vi "Wind_Turbine.vi"() -> (5 "Plug in titles":string[](array[string]), 7 "Plug in values":string[](array[string]))   [LabVIEW 2013]
uses:
  <vilib>/Analysis/baseanly.llb/Mean (DBL).vi
  Globals/Meas_global.vi
  Globals/LDA_meas_global_1.vi
  <vilib>/Analysis/NI_AALBase.lvlib
  <vilib>/Analysis/NI_AALPro.lvlib
panel:
  in  "Time Shift":dbl
  out "X array":dbl[](array[numeric])
  out "WT Numbers":string[](array[string])
  out "WT Revolution Start times":dbl[](array[numeric])
  out "Laser Disp Index":i32
  out "Laser Phase lock index":i32
  out "Laser Status Index":i32
  out "L Status Phase lock index":i32
  in  "Tab Control":T1(tab)
  in  "Change Dem Voltages?":bool=TRUE
  in  "Allow large changes?":bool
  out "Turbine RPMs":cluster{i32[], "All WTs":dbl[]}(graph)
  out "All WTs":dbl[][](array[numeric]) format="%#.2g"
  out "Cross Chs":cluster{dbl[], dbl[]}[](graph)
  in  "Cross_Corr to Phase Lock":i32[](listbox)
  in  "Channel to Phase lock":i32[](listbox)
  in  "Turbine to Phase Lock to":u16(ring) items=["RV (WT1)"]
  out "Inst Channels":cluster{dbl[], dbl[]}[](graph)
  in  "Add Phase data to results file":bool
  in  "Save Phase averaged Profiles":bool
  in  "Output Directory":path
  in  "Separation Character":string="\t"
  in  "Angular Step":dbl=1.0
  in  "Precision":string
  out "Av Disp 1":dbl
  out "Av Disp 2":dbl
  out "Av Disp 3":dbl
  out "Av Variance 1":dbl
  out "Av Variance 2":dbl
  out "Av Variance 3":dbl
  out "Angle 1":dbl format="%#_3g"
  out "Angle 2":dbl format="%#_3g"
  out "Angle 3":dbl format="%#_3g"
  out "Mean Blade 1":cluster{dbl, "Angular Step":dbl, dbl[]}(graph)
  out "slope 1":dbl format="%#_3g"
  out "Mean Blade 2":cluster{dbl, "Angular Step":dbl, dbl[]}(graph)
  out "Mean Blade 3":cluster{dbl, "Angular Step":dbl, dbl[]}(graph)
  out "slope 2":dbl format="%#_3g"
  out "slope 3":dbl format="%#_3g"
  out "Blade Positions":dbl[][](graph)
  out "Blade Angles":dbl[][](graph)
  out "Blade 1 Every Pass":dbl[](graph)
  out "Blade 2 Every Pass":dbl[](graph)
  out "Blade 3 Every Pass":dbl[](graph)
  out "Blade Analysis":string[][](table)
  in  "End Cut Deg":dbl
  in  "Start Cut Deg":dbl
  # "Mean RPM      SD RPM           Max-Min"
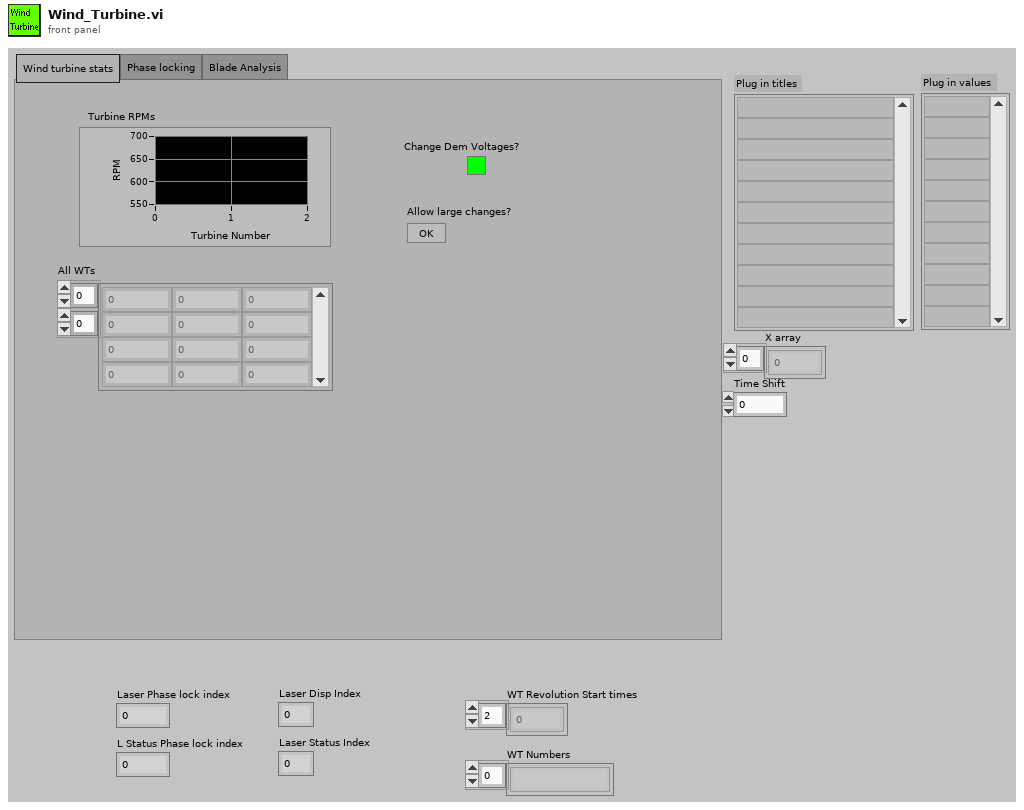
[diagram p1: front panel]
types:
  T1 = enum32{"Wind turbine stats", "Phase locking", "Blade Analysis"}
  T2 = typedef "Post_Process.ctl" = enum16{"Take New Data", "Post Process Raw Data File"}
  T3 = typedef "Analysis_info_cluster.ctl" = cluster{"Colour":u32, "Inst type":T4, "Inst name":string, "Symbol":string, "Code name":string, "Extra Info":string, "Inst Array":T5, "Extra Titles":string[], "Extra Values":string[], "U":dbl, "u^2":dbl, "u^3":dbl, "u^4":dbl, "Skew_u":dbl, "Kurt_u":dbl, "Sd Error in Mean":dbl, "% u'/U":dbl, "X":dbl, "Y":dbl, "Z":dbl, "Timescale integral to 25%":dbl, "Sd Error in Variance":dbl, "Calib File":path, "Calib Constants":dbl[], "Output Position":bool, "Full Stats":bool, "Av Sampling Rate":dbl, "Av No of Samples":dbl, "Total Meas Time (s)":dbl, "ADAM Ch Name":string}
  T4 = typedef "Inst_type.ctl" = enum16{"Propeller anemometer", "Raw voltage", "Pressure Transducer", "Pitot-static tube", "Preston tube", "Hot wire", "Cross wire 1", "Cross wire 2", "Generic Linear", "Generic Polynomial", "Generic BackPoly", "Fast FID", "Thermocouple", "Cold wire", "Pulsed Wire", "LDA Vel", "LDA Tran time", "LDA Arr time"}
  T5 = typedef "Instrument_Array.ctl" = enum16{"PWA", "LDA", "Analogue"}
  T6 = typedef "Time_Trace_Cluster.ctl" = cluster{"Weighting":dbl[], "Time (s)":dbl[], "Voltage":dbl[], "Eng Values":dbl[]}
  T7 = cluster{"X array":dbl[], "Phase locked uw/u'w'":dbl[]}
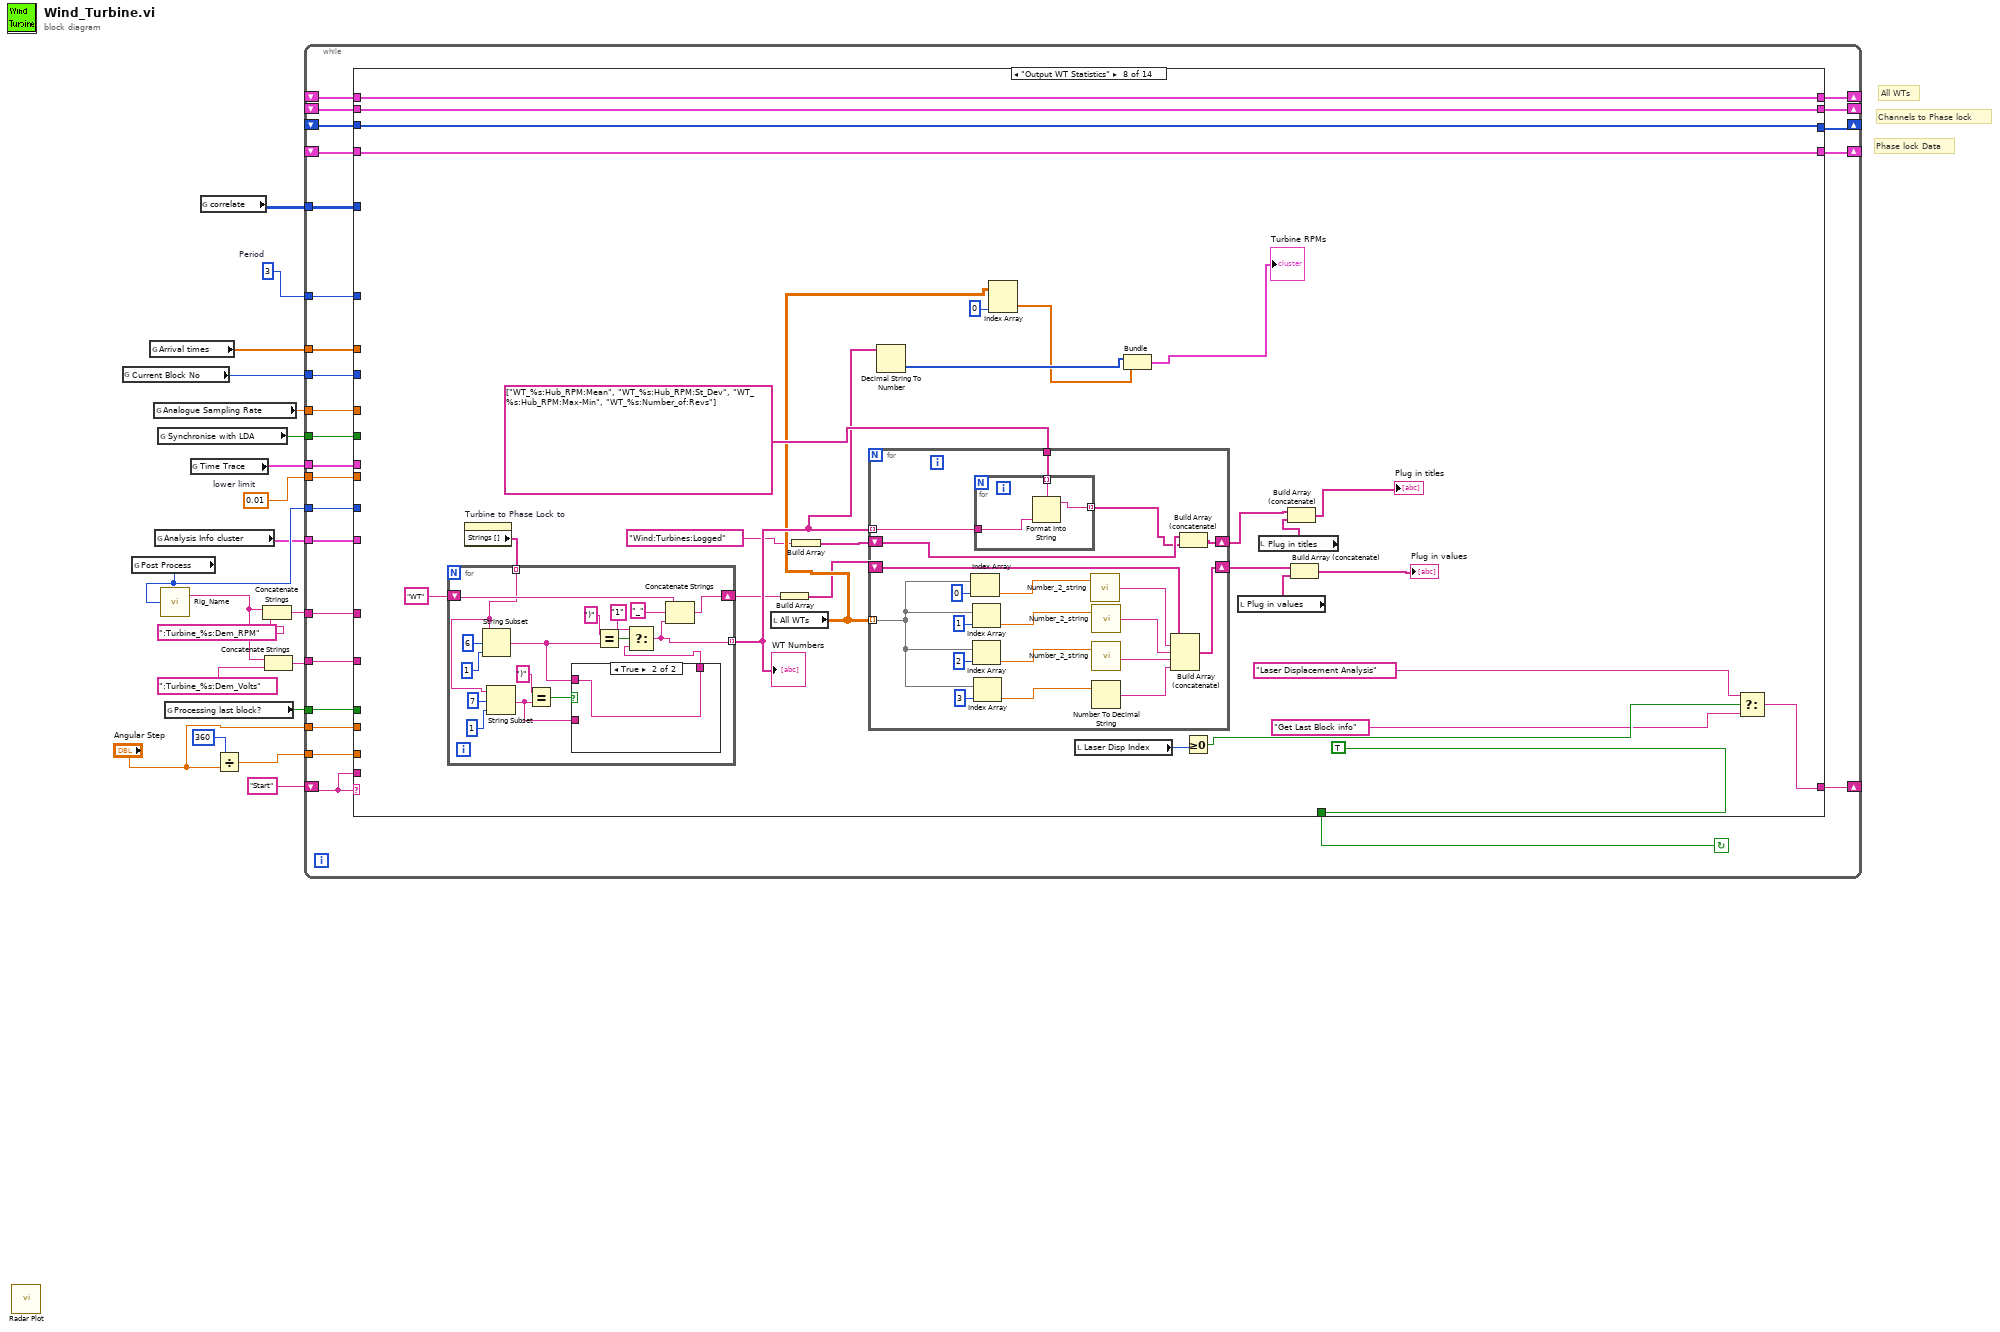
[diagram p0: block diagram]
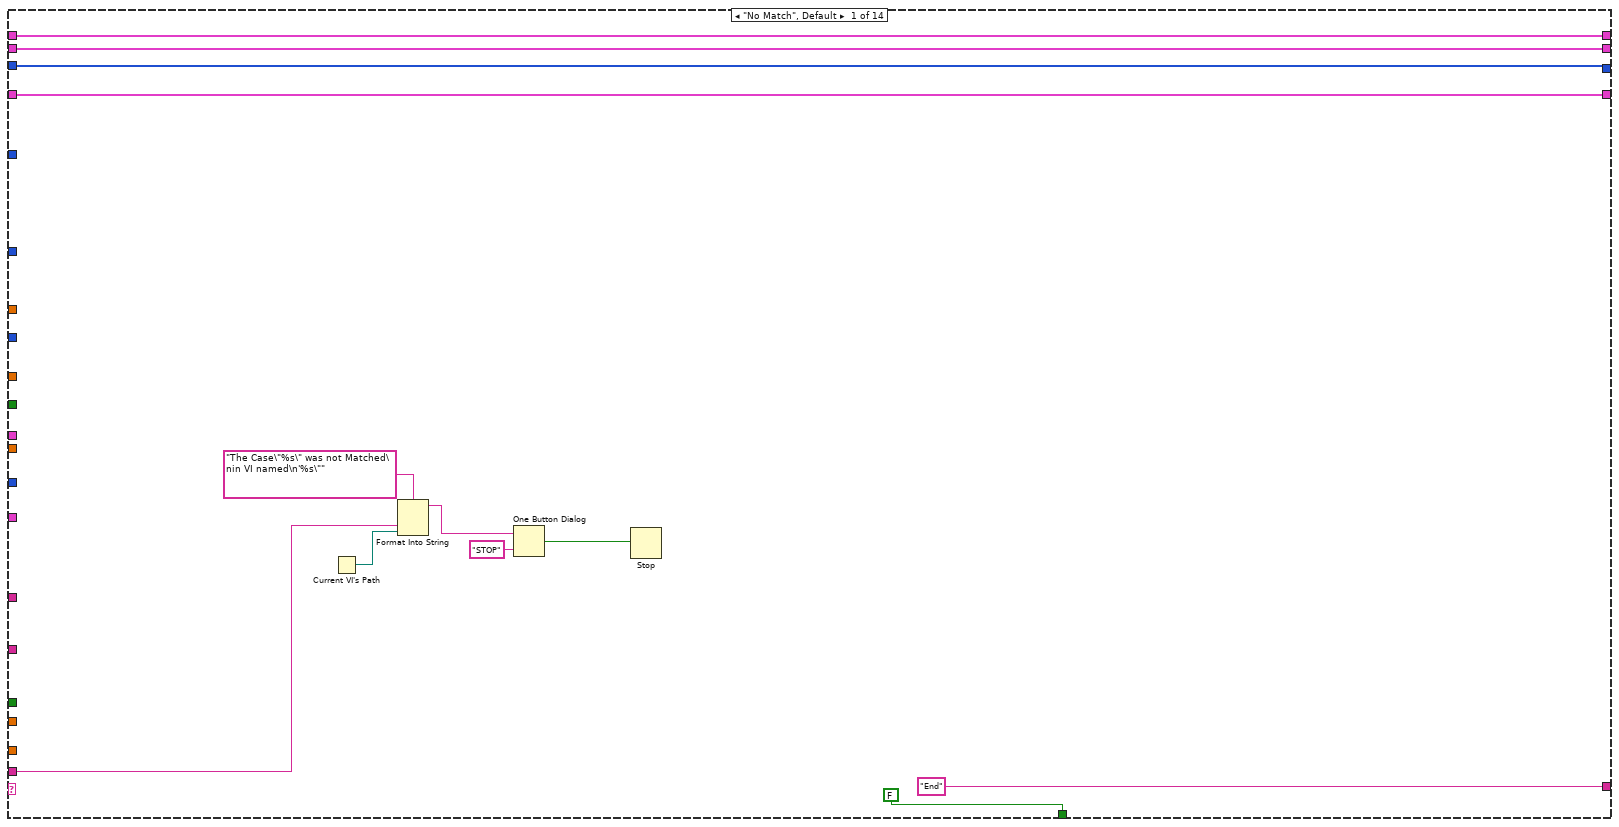
[diagram p2: hidden frame]
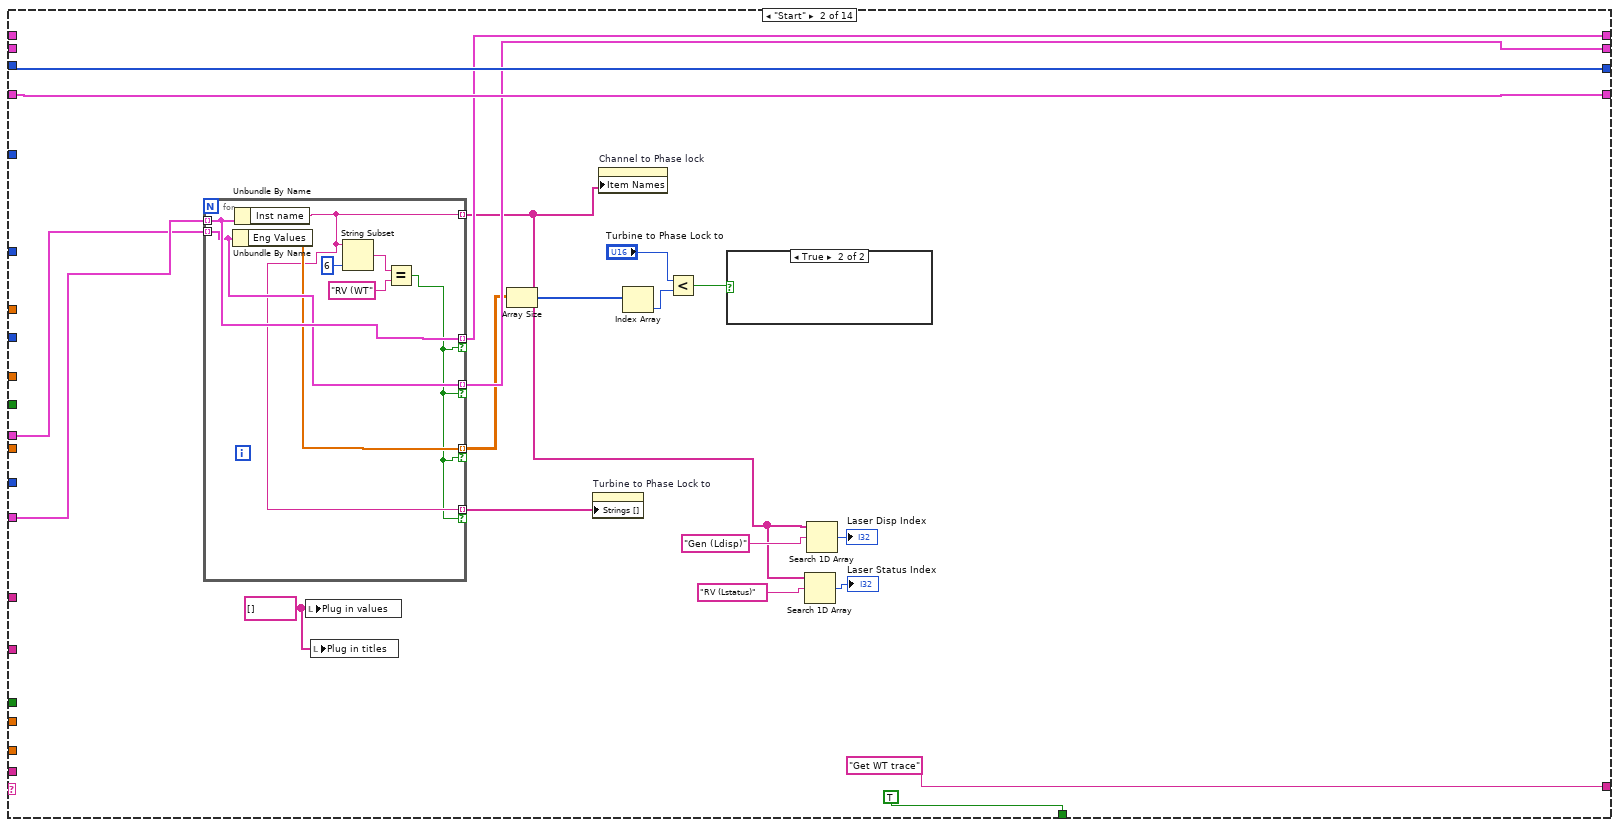
[diagram p3: hidden frame]
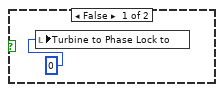
[diagram p4: hidden frame]
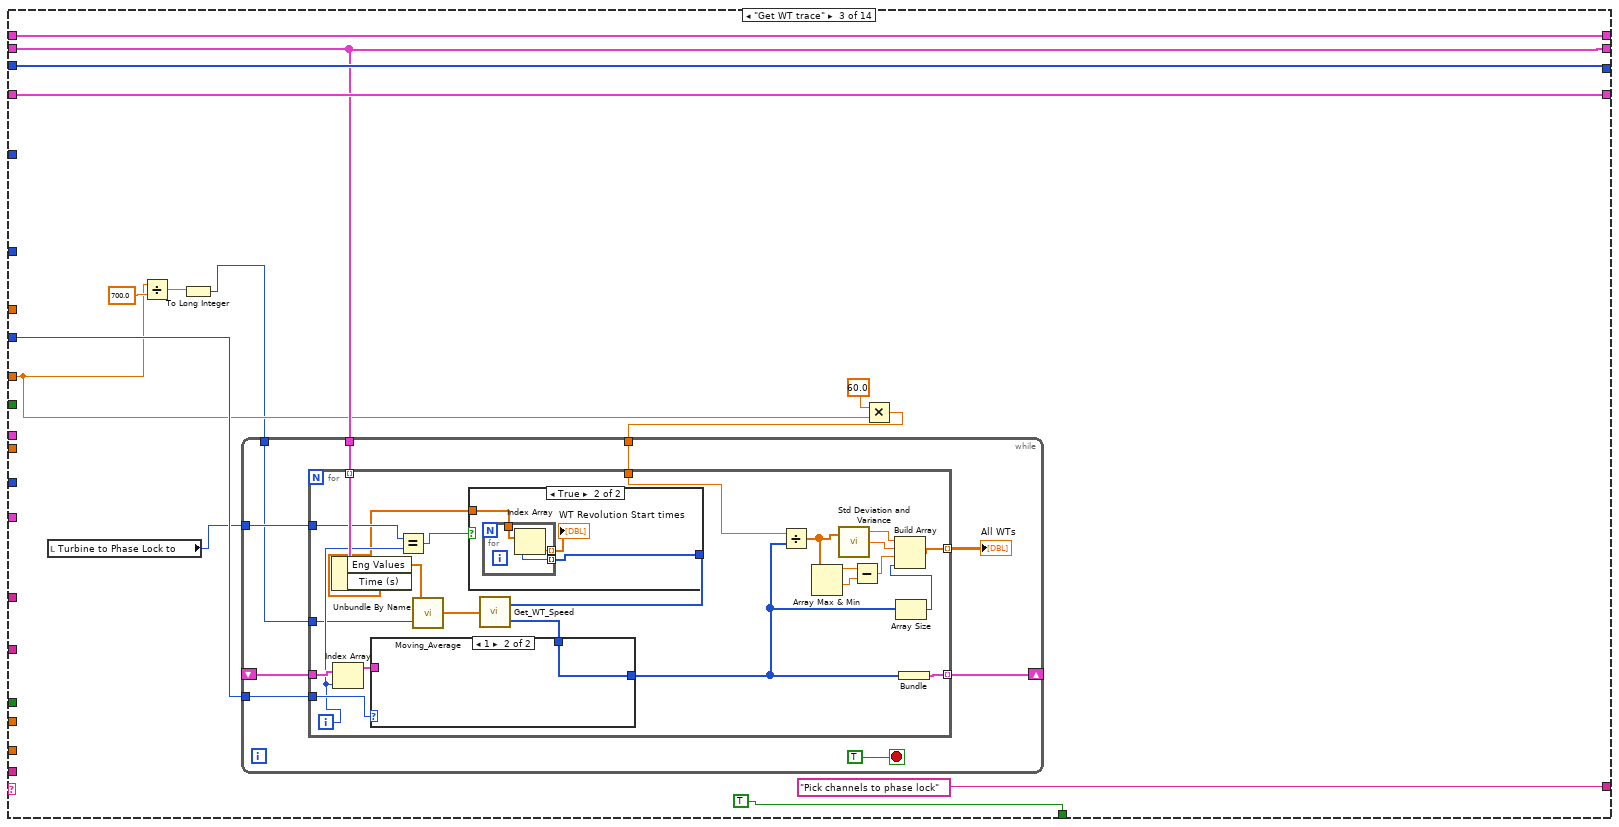
[diagram p5: hidden frame]
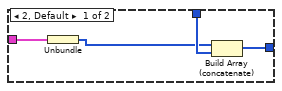
[diagram p7: hidden frame]
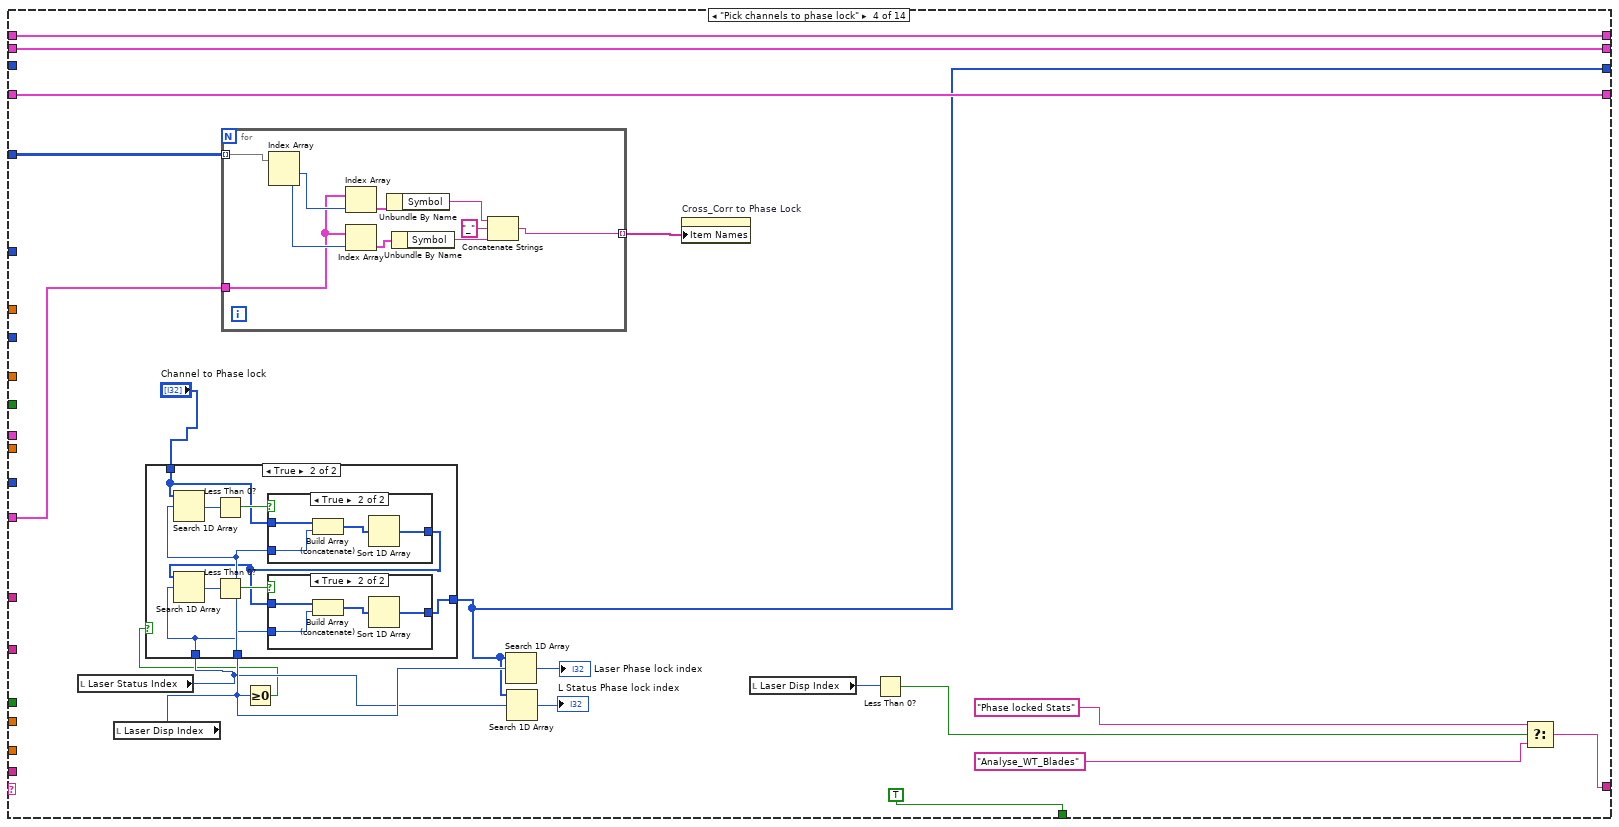
[diagram p8: hidden frame]
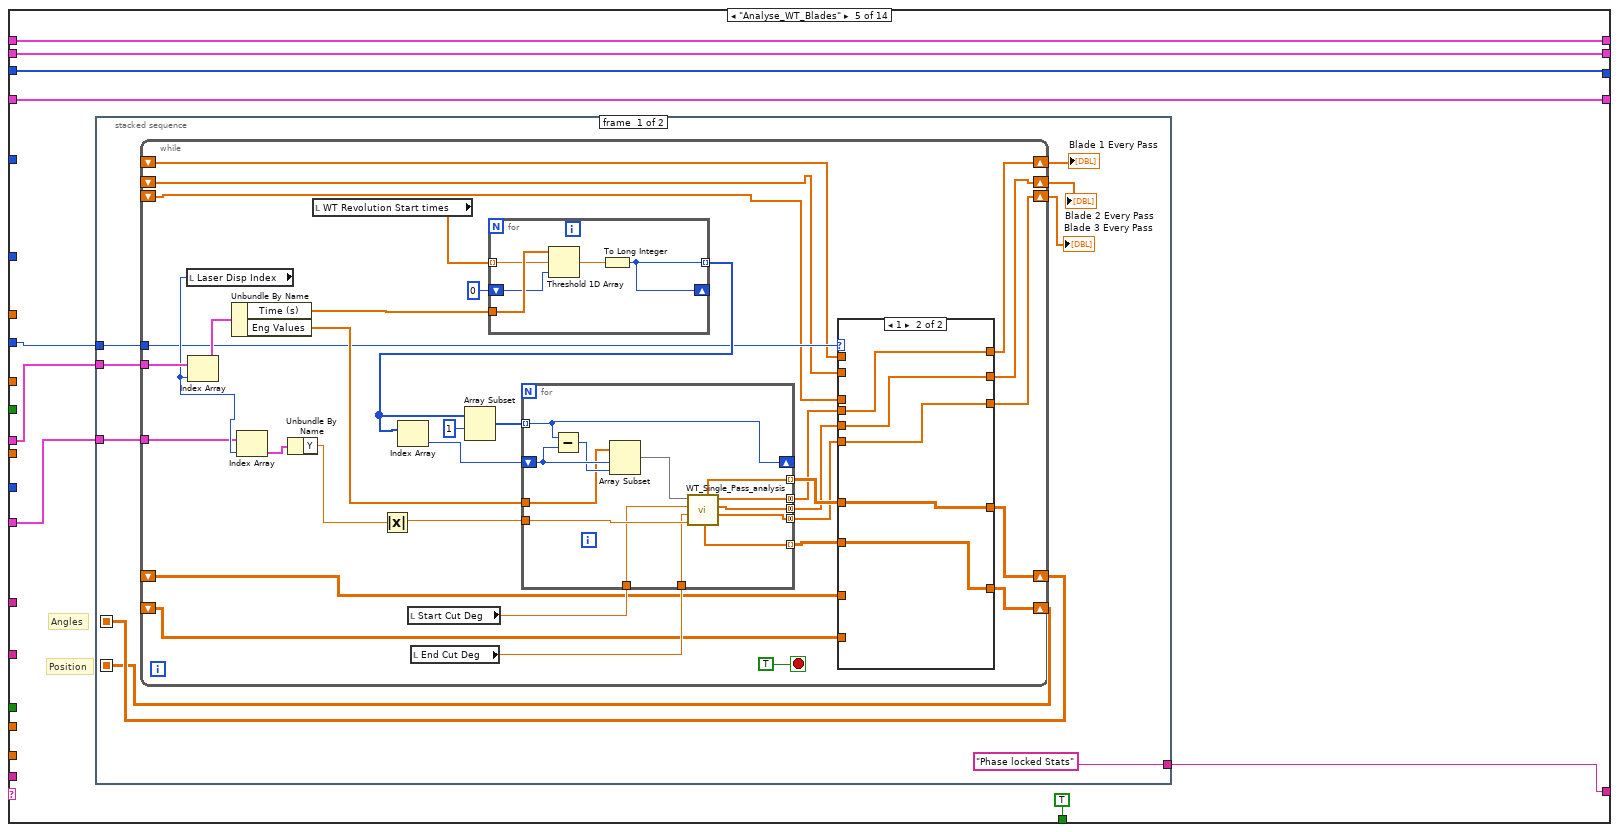
[diagram p12: hidden frame]
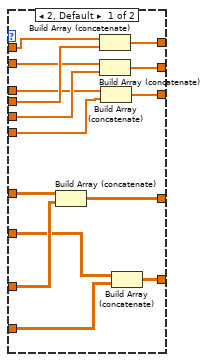
[diagram p13: hidden frame]
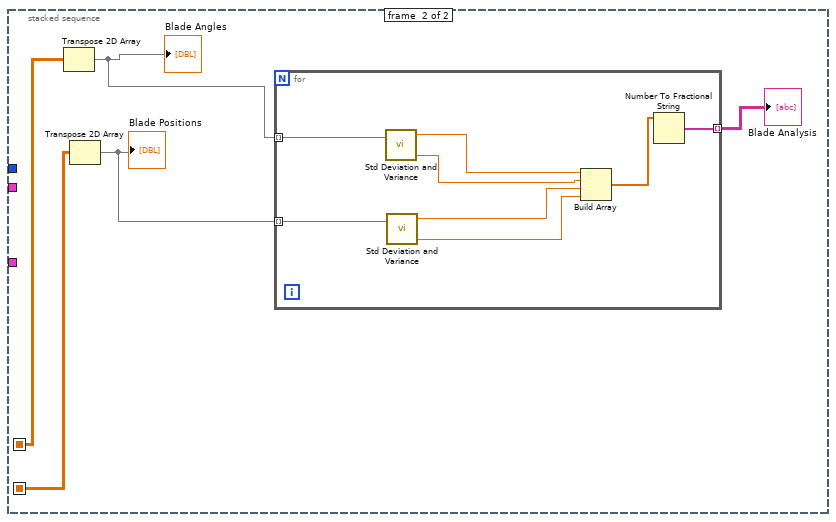
[diagram p14: hidden frame]
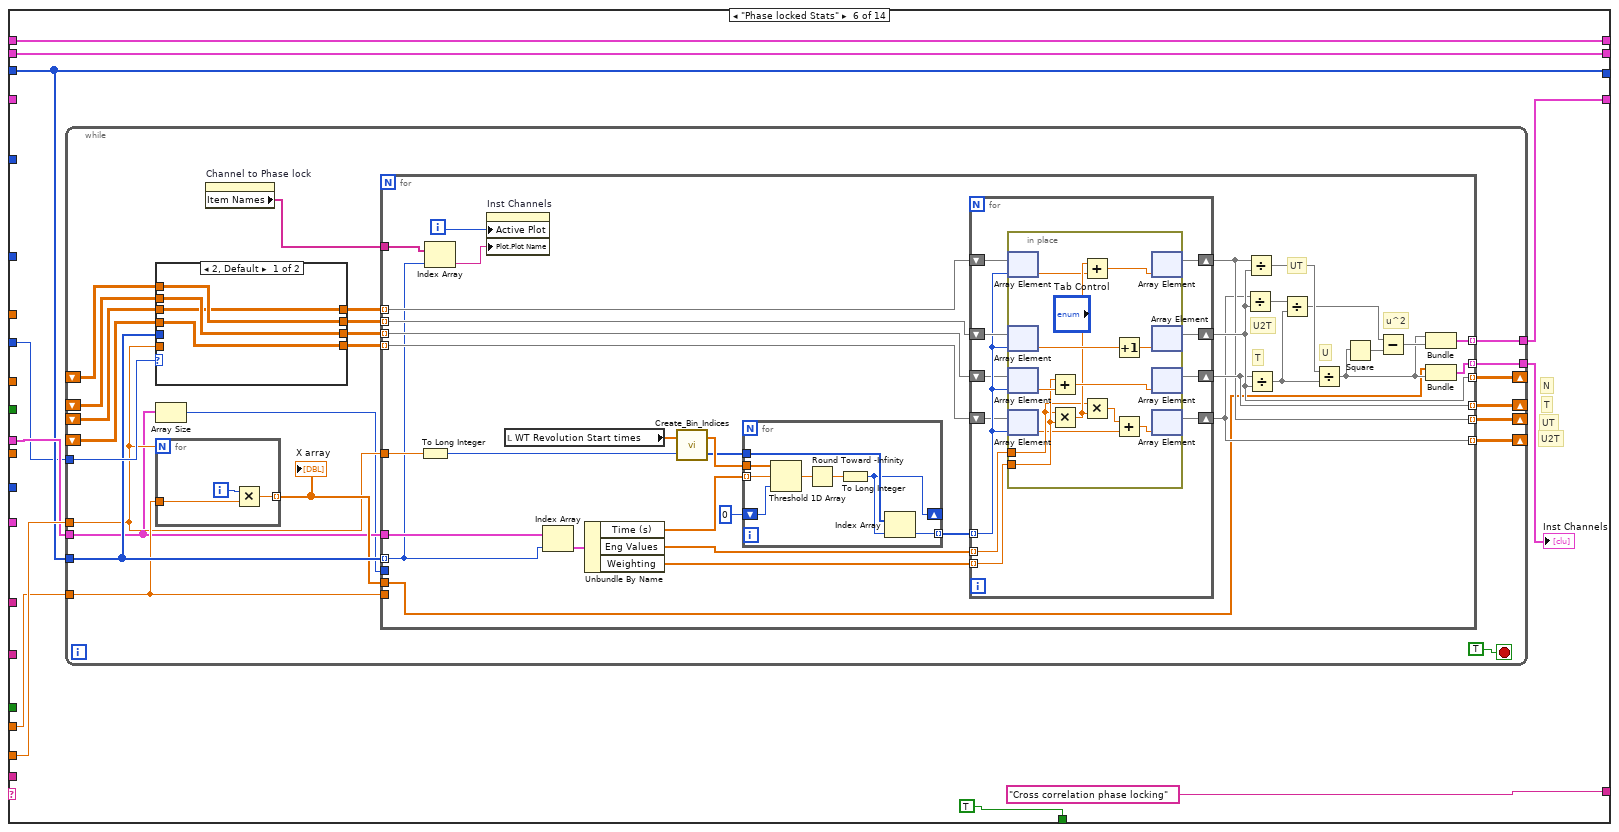
[diagram p15: hidden frame]
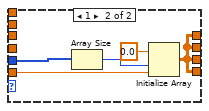
[diagram p16: hidden frame]
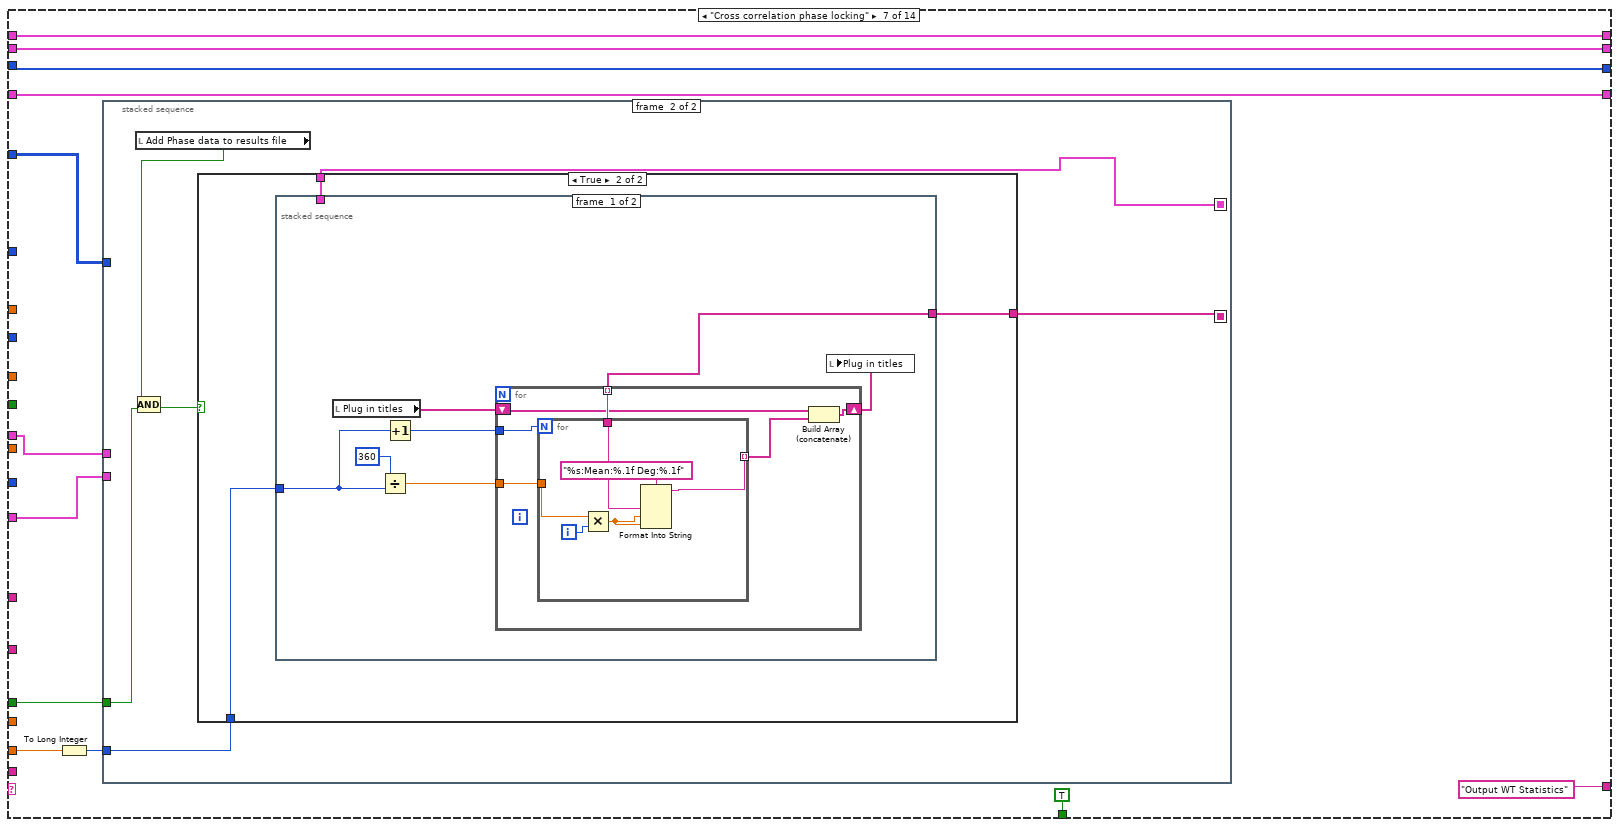
[diagram p17: hidden frame]
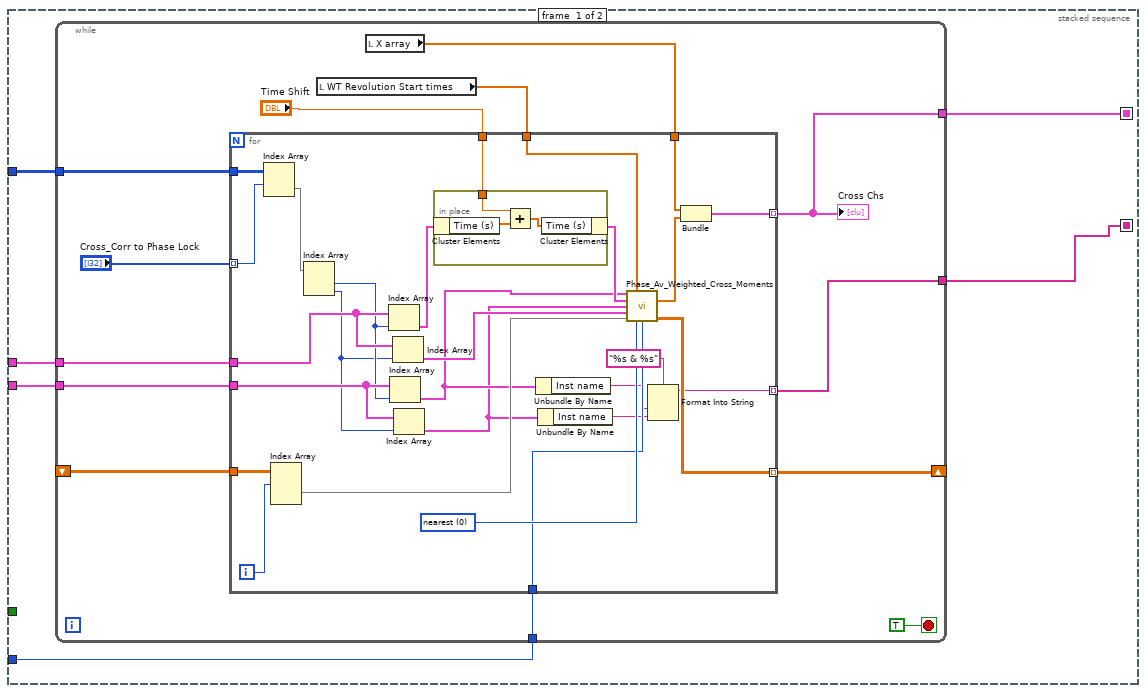
[diagram p18: hidden frame]
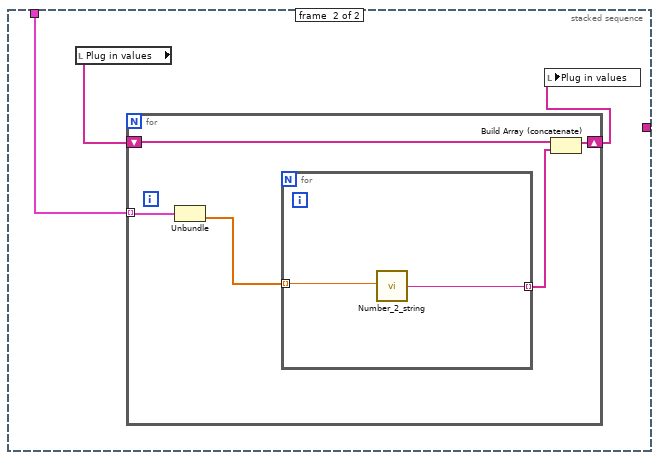
[diagram p20: hidden frame]
diagram:
  w18 = 3  # Period
  w19 = 0.01  # lower limit
  # "Phase lock Data"
  # "Channels to Phase lock"
  # "All WTs"
  n1 = call <vilib>:"Radar Plot.vi"() -> ()  [unwired: 15 in, 1 out]
  n2 = global read "Meas_global.vi" "Current Block No"() -> (w5:i32)
  n3 = global read "Meas_global.vi" "Post Process"() -> (w17:T2)
  n4 = global read "LDA_meas_global_1.vi" "Arrival times"() -> (w8:dbl[])
  n5 = global read "Meas_global.vi" "Analogue Sampling Rate"() -> (w20:dbl)
  n6 = global read "Meas_global.vi" "Analysis Info cluster"() -> (w7:T3[])
  n7 = global read "Meas_global.vi" "Synchronise with LDA"() -> (w12:bool)
  n8 = call "Rig_Name.vi"("Post Process"=w17) -> ("Rig Setup before dash"=w14:string)  [unwired: 1 out]
  n9 = global read "Meas_global.vi" "Processing last block?"() -> (w10:bool)
  n10 = global read "Meas_global.vi" "Time Trace"() -> (w3:T6[])
  n11 = global read "Meas_global.vi" "correlate"() -> (w1:i32[][])
  n12 = Divide(x=360, y="Angular Step") -> (x/y=w6:dbl)
  n13 = Concatenate Strings(w14, ":Turbine_%s:Dem_RPM") -> (w13:string)
  n14 = Concatenate Strings(w14, ":Turbine_%s:Dem_Volts") -> (w16:string)
  n15 = while {
    tunnel: w5 -> [w46]
    tunnel: w20 -> [w45]
    tunnel: w16 -> [w44]
    tunnel: w13 -> [w43]
    tunnel: w19 -> [w42]
    tunnel: w18 -> [w41]
    tunnel: w17 -> [w40]
    tunnel: w12 -> [w39]
    tunnel: w7 -> [w38]
    shift-right: [w22] -> _
    shift-left: "Start" -> [w36]
    tunnel: w10 -> [w35]
    tunnel: w6 -> [w34]
    tunnel: w8 -> [w33]
    tunnel: "Angular Step" -> [w32]
    shift-right: [w31] -> _
    shift-left: _ -> [w30]
    shift-right: [w28] -> _
    shift-left: _ -> [w29]
    shift-right: [w27] -> _
    shift-left: _ -> [w26]
    tunnel: w3 -> [w25]
    shift-right: [w24] -> _
    shift-left: _ -> [w23]
    tunnel: w1 -> [w21]
    stop <- w37 continue-if-true
    n16 = case shown="\"Output WT Statistics\"" w36 {
      tunnel: w46 -> [_ _ w97 _ w196 w301 _ _ _ _ _ _ _ _]
      tunnel: w45 -> [_ _ w90 _ _ _ _ _ w591 _ _ _ _ w975]
      tunnel: w44 -> [_ _ _ _ _ _ _ _ _ _ w865 _ _ _]
      tunnel: w43 -> [_ _ _ _ _ _ _ _ _ _ w840 _ _ _]
      tunnel: w42 -> [_ _ _ _ _ _ _ _ _ _ _ _ _ _]
      tunnel: w41 -> [_ _ _ _ _ _ _ _ _ _ _ _ _ _]
      tunnel: w40 -> [_ _ _ _ _ _ _ _ _ w825 _ _ _ _]
      tunnel: w39 -> [_ _ _ _ _ _ _ _ _ _ _ _ _ _]
      tunnel: w38 -> [_ w78 _ w148 w198 _ w412 _ w581 _ _ _ _ _]
      tunnel: ["End" "Get WT trace" "Pick channels to phase lock" w149 w195 "Cross correlation phase locking" "Output WT Statistics" w532 w586 w824 "End" ("f") "Check Folder Name" "Save Phase locked data" "End"] -> w22
      tunnel: [FALSE ("Change Control Voltage?") TRUE ("Processing last block?") TRUE TRUE ("Change Control Voltage?") TRUE ("Change Control Voltage?") TRUE TRUE ("Change Control Voltage?") TRUE ("Change Control Voltage?") w587 w823 FALSE ("Change Control Voltage?") w901 w952 FALSE ("Change Control Voltage?")] -> w37
      tunnel: w36 -> [w53 _ _ _ _ _ _ _ _ _ _ _ _ _]
      tunnel: w35 -> [_ _ _ _ _ _ w409 _ w588 w822 _ w899 _ _]
      tunnel: w34 -> [_ _ _ _ _ w308 w411 _ w590 _ _ w897 _ _]
      tunnel: w33 -> [_ _ _ _ _ _ _ _ _ _ _ _ _ _]
      tunnel: w32 -> [_ _ _ _ _ w307 _ _ w589 _ _ _ _ w969]
      tunnel: [w50 w64 w93 w164 w203 w306 w418 w529 w585 w821 w839 w896 w950 w972] -> w31
      tunnel: w30 -> [w50 _ w93 w164 w203 w306 w418 w529 w585 w821 w839 w896 w950 w972]
      tunnel: w29 -> [w49 w65 w95 _ w201 w302 w416 w528 w584 w820 w838 w895 w949 w971]
      tunnel: [w49 w65 w95 w155 w201 w302 w416 w528 w584 w820 w838 w895 w949 w971] -> w28
      tunnel: [w48 w66 w94 w159 w200 w300 w415 w527 w582 w819 w837 w893 w948 w970] -> w27
      tunnel: w26 -> [w48 w66 w94 w159 w200 _ w415 w527 w582 w819 w837 w893 w948 w970]
      tunnel: w25 -> [_ w67 _ _ w199 w303 w413 _ _ _ _ _ _ _]
      tunnel: [w47 w63 w92 w158 w202 w304 w417 w526 w583 w818 w836 w894 w947 w968] -> w24
      tunnel: w23 -> [w47 _ w92 w158 w202 w304 w417 w526 w583 w818 w836 w894 w947 w968]
      tunnel: w21 -> [_ _ _ w146 _ _ w414 _ _ _ _ _ _ _]
      frame "No Match", Default {
        n17 = Current VI's Path() -> (path=w54:path)
        n18 = Format Into String(format string="The Case\"%s\" was not Matched\nin VI named\n'%s\"" ("Format String"), w53, w54) -> (resulting string=w57:string)  [unwired: 2 in, 1 out]
        n19 = One Button Dialog(message=w57, button name ("OK")="STOP") -> (true=w55:bool)
        n20 = Stop(stop? (T)=w55) -> ()
      }
      frame "Start" {
        w59 = string[] [] ("Plug in values")
        n21 = for {
          tunnel: w78 -> [w84] mode=indexing
          tunnel: [w81] -> w60 mode=indexing
          tunnel: w67 -> [w83] mode=indexing
          tunnel: [w84] -> w64 mode=indexing if=w80
          tunnel: [w83] -> w63 mode=indexing if=w80
          tunnel: [w82] -> w62 mode=indexing if=w80
          tunnel: [w81] -> w61 mode=indexing if=w80
          n22 = Unbundle By Name(w83) -> ("Eng Values"=w82:dbl[])
          n23 = Unbundle By Name(w84) -> ("Inst name"=w81:string)
          n24 = String Subset(string=w81, length (rest)=6 ("length (rest)")) -> (substring=w85:string)  [unwired: 1 out]
          n25 = Equal?(x=w85, y="RV (WT") -> (x = y?=w80:bool)
        }
        n26 = local write "Plug in values"(w59) -> ()
        n27 = local write "Plug in titles"(w59) -> ()
        n28 = Array Size(array=w62) -> (size(s)=w69:i32[])
        n29 = property on="Turbine to Phase Lock to" class="Ring (strict)"("Strings []"=w61) -> ()  [unwired: 2 in, 2 out]
        n30 = property on="Channel to Phase lock" class="LstBox (strict)"("Item Names"=w60) -> ()  [unwired: 2 in, 2 out]
        n31 = Index Array(array=w69) -> (element=w68:i32)  [unwired: 1 in]
        n32 = Less?(x="Turbine to Phase Lock to", y=w68) -> (x < y?=w74:bool)
        n33 = case shown="True" w74 {
          frame False {
            n34 = local write "Turbine to Phase Lock to"(0) -> ()
          }
          frame True {
          }
        }
        n35 = Search 1D Array(1D array=w60, element="RV (Lstatus)") -> (index of element=→"Laser Status Index":i32)  [unwired: 1 in]
        n36 = Search 1D Array(1D array=w60, element="Gen (Ldisp)") -> (index of element=→"Laser Disp Index":i32)  [unwired: 1 in]
      }
      frame "Get WT trace" {
        n37 = local read "Turbine to Phase Lock to"() -> (w96:u16)
        n38 = Divide(x=w90, y=700.0) -> (x/y=w89:dbl)
        n39 = To Long Integer(number=w89) -> (32bit integer=w88:i32)
        n40 = Multiply(x=60.0, y=w90) -> (x*y=w98:dbl)
        n41 = while {
          tunnel: w97 -> [w110]
          shift-right: [w105] -> _
          shift-left: _ -> [w109]
          tunnel: w98 -> [w108]
          tunnel: w92 -> [w104]
          tunnel: w96 -> [w103]
          tunnel: w88 -> [w102]
          stop <- TRUE stop-if-true
          n42 = for {
            tunnel: w110 -> [w133]
            tunnel: w109 -> [w123]
            tunnel: w108 -> [w131]
            tunnel: [w124] -> w106 mode=indexing
            tunnel: [w119] -> w105 mode=indexing
            tunnel: w104 -> [w118] mode=indexing
            tunnel: w103 -> [w114]
            tunnel: w102 -> [w111]
            i -> [w115]
            n43 = Unbundle By Name(w118) -> ("Eng Values"=w117:dbl[], "Time (s)"=w112:dbl[])
            n44 = Index Array(array=w123, index=w115) -> (element=w122:cluster{"Samples per pulse":i32[]})
            n45 = Equal?(x=w114, y=w115) -> (x = y?=w113:bool)
            n46 = call "Moving_Average.vi"("Period"=w111, "Input Array"=w117) -> ("N+1-Period"=w134:dbl[])
            n47 = call "Get_WT_Speed.vi"("Opto Trace"=w134) -> ("Start Cycle Index"=w116:i32[], "Samples per pulse"=w132:i32[])
            n48 = case shown="1" w133 {
              tunnel: [w143 w145] -> w120
              tunnel: w132 -> [w144 w145]
              tunnel: w122 -> [w142 _]
              frame 2, Default {
                n49 = Unbundle(w142) -> ("Samples per pulse"=w141:i32[])
                n50 = Build Array (concatenate)(w141, w144) -> (w143:i32[])
              }
              frame 1 {
              }
            }
            n51 = case shown="True" w113 {
              tunnel: w116 -> [_ w137]
              tunnel: w112 -> [_ w136]
              frame False {
              }
              frame True {
                n52 = for {
                  tunnel: w137 -> [w140] mode=indexing
                  tunnel: w136 -> [w139]
                  tunnel: [w138] -> w135 mode=indexing
                  n53 = Index Array(array=w139, index=w140) -> (element=w138:dbl)
                }
                "WT Revolution Start times" <- w135
              }
            }
            n54 = Divide(x=w131, y=w120) -> (x/y=w128:dbl[])
            n55 = Array Max & Min(array=w128) -> (max value=w130:dbl, min value=w129:dbl)  [unwired: 2 out]
            n56 = call <vilib>:"Std Deviation and Variance.vi"("X"=w128) -> ("mean"=w127:dbl, "standard deviation"=w126:dbl)  [unwired: 1 in, 1 out]
            n57 = Subtract(x=w130, y=w129) -> (x-y=w125:dbl)
            n58 = Array Size(array=w120) -> (size(s)=w121:i32)
            n59 = Build Array(w127, w126, w125, w121) -> (w124:dbl[])
            n60 = Bundle("Samples per pulse"=w120) -> (w119:cluster{"Samples per pulse":i32[]})  [unwired: 1 in]
          }
          "All WTs" <- w106
        }
      }
      frame "Pick channels to phase lock" {
        n61 = local read "Laser Status Index"() -> (w161:i32)
        n62 = local read "Laser Disp Index"() -> (w162:i32)
        n63 = for {
          tunnel: w146 -> [w174] mode=indexing
          tunnel: w148 -> [w171]
          tunnel: [w165] -> w147 mode=indexing
          n64 = Index Array(array=w174) -> (element #1=w173:i32, element #2=w172:i32)  [unwired: 2 in]
          n65 = Index Array(array=w171, index=w173) -> (element=w170:T3)
          n66 = Index Array(array=w171, index=w172) -> (element=w169:T3)
          n67 = Unbundle By Name(w170) -> ("Symbol"=w168:string)
          n68 = Unbundle By Name(w169) -> ("Symbol"=w167:string)
          n69 = Concatenate Strings(w168, "_" ("string"), w167) -> (w165:string)
        }
        n70 = Greater Or Equal To 0?(x=w162) -> (x >= 0?=w160:bool)
        n71 = case shown="True" w160 {
          tunnel: "Channel to Phase lock" -> [w175 w182]
          tunnel: w162 -> [_ w181]
          tunnel: [w175 w178] -> w155
          tunnel: w161 -> [_ w176]
          frame False {
          }
          frame True {
            n72 = Search 1D Array(1D array=w182, element=w181) -> (index of element=w184:i32)  [unwired: 1 in]
            n73 = Less Than 0?(x=w184) -> (x < 0?=w183:bool)
            n74 = case shown="True" w183 {
              tunnel: w182 -> [w190 w194]
              tunnel: w181 -> [_ w193]
              tunnel: [w190 w191] -> w177
              frame False {
              }
              frame True {
                n75 = Build Array (concatenate)(w194, w193) -> (w192:i32[])
                n76 = Sort 1D Array(array=w192) -> (sorted array=w191:i32[])
              }
            }
            n77 = Search 1D Array(1D array=w177, element=w176) -> (index of element=w179:i32)  [unwired: 1 in]
            n78 = Less Than 0?(x=w179) -> (x < 0?=w180:bool)
            n79 = case shown="True" w180 {
              tunnel: w177 -> [w185 w189]
              tunnel: w176 -> [_ w188]
              tunnel: [w185 w186] -> w178
              frame False {
              }
              frame True {
                n80 = Build Array (concatenate)(w189, w188) -> (w187:i32[])
                n81 = Sort 1D Array(array=w187) -> (sorted array=w186:i32[])
              }
            }
          }
        }
        n82 = Search 1D Array(1D array=w155, element=w162) -> (index of element=→"Laser Phase lock index":i32)  [unwired: 1 in]
        n83 = Search 1D Array(1D array=w155, element=w161) -> (index of element=→"L Status Phase lock index":i32)  [unwired: 1 in]
        n84 = property on="Cross_Corr to Phase Lock" class="LstBox (strict)"("Item Names"=w147) -> ()  [unwired: 2 in, 2 out]
        n85 = local read "Laser Disp Index"() -> (w153:i32)
        n86 = Less Than 0?(x=w153) -> (x < 0?=w152:bool)
        n87 = Select(t="Phase locked Stats" ("f"), s=w152, f="Analyse_WT_Blades") -> (s? t:f=w149:string)
      }
      frame "Analyse_WT_Blades" {
        # "Position"
        # "Angles"
        n88 = stacked-sequence {
          seq-local: [w207 _] -> [_ w288]
          seq-local: [w208 _] -> [_ w289]
          tunnel: w199 -> [w212 _]
          tunnel: w198 -> [w211 _]
          tunnel: w196 -> [w210 _]
          tunnel: ["Phase locked Stats" ("f") _] -> w195
          frame #0 {
            n89 = while {
              tunnel: w212 -> [w246]
              tunnel: w211 -> [w235]
              shift-right: [w225] -> w208
              shift-left: _ -> [w226]
              shift-right: [w222] -> w207
              shift-left: _ -> [w223]
              tunnel: w210 -> [w228]
              shift-right: [w220] -> w206
              shift-left: _ -> [w219]
              shift-right: [w215] -> w205
              shift-left: _ -> [w216]
              shift-right: [w213] -> w204
              shift-left: _ -> [w214]
              stop <- TRUE stop-if-true
              n90 = local read "Laser Disp Index"() -> (w236:i32)
              n91 = Index Array(array=w246, index=w236) -> (element=w245:T6)
              n92 = Unbundle By Name(w245) -> ("Time (s)"=w244:dbl[], "Eng Values"=w237:dbl[])
              n93 = Index Array(array=w235, index=w236) -> (element=w234:T3)
              n94 = Unbundle By Name(w234) -> ("Y"=w233:dbl)
              n95 = local read "WT Revolution Start times"() -> (w243:dbl[])
              n96 = Absolute Value(x=w233) -> (abs(x)=w232:dbl)
              n97 = local read "Start Cut Deg"() -> (w231:dbl)
              n98 = local read "End Cut Deg"() -> (w230:dbl)
              n99 = for {
                tunnel: w244 -> [w284]
                tunnel: w243 -> [w283] mode=indexing
                shift-right: [w280] -> _
                shift-left: 0 -> [w282]
                tunnel: [w280] -> w240 mode=indexing
                n100 = Threshold 1D Array(1:w282, 2:w283, 3:w284) -> (0:w281:dbl)
                n101 = To Long Integer(number=w281) -> (32bit integer=w280:i32)
              }
              n102 = Index Array(array=w240) -> (element=w239:i32)  [unwired: 1 in]
              n103 = Array Subset(array=w240, index=1) -> (w238:i32[])  [unwired: 1 in]
              n104 = for {
                shift-right: [w278] -> _
                shift-left: w239 -> [w279]
                tunnel: w238 -> [w278] mode=indexing
                tunnel: w237 -> [w276]
                tunnel: w232 -> [w274]
                tunnel: [w270] -> w227 mode=indexing
                tunnel: [w273] -> w224 mode=indexing
                tunnel: w231 -> [w272]
                tunnel: w230 -> [w271]
                tunnel: [w269] -> w221 mode=concatenating
                tunnel: [w268] -> w218 mode=concatenating
                tunnel: [w267] -> w217 mode=concatenating
                n105 = Subtract(x=w278, y=w279) -> (x-y=w277:i32)
                n106 = Array Subset(array=w276, index=w279, length=w277) -> (w275:dbl[])
                n107 = call "WT_Single_Pass_analysis.vi"("Displacement"=w275, "Start Cut Deg"=w272, "End Cut Deg"=w271, "Radius"=w274) -> ("Blade Angles"=w270:dbl[], "Blade Positions"=w273:dbl[], "Blade1"=w269:dbl[], "Blade 2"=w268:dbl[], "Blade 3"=w267:dbl[])  [unwired: 1 in]
              }
              n108 = case shown="1" w228 {
                tunnel: w227 -> [w261 w266]
                tunnel: w226 -> [w260 _]
                tunnel: [w259 w266] -> w225
                tunnel: w224 -> [w258 w265]
                tunnel: w223 -> [w257 _]
                tunnel: [w256 w265] -> w222
                tunnel: w221 -> [w255 w264]
                tunnel: [w253 w264] -> w220
                tunnel: w219 -> [w254 _]
                tunnel: w218 -> [w252 w263]
                tunnel: w217 -> [w251 w262]
                tunnel: w216 -> [w250 _]
                tunnel: [w249 w263] -> w215
                tunnel: w214 -> [w248 _]
                tunnel: [w247 w262] -> w213
                frame 2, Default {
                  n109 = Build Array (concatenate)(w261, w260) -> (w259:dbl[][])
                  n110 = Build Array (concatenate)(w254, w255) -> (w253:dbl[])
                  n111 = Build Array (concatenate)(w250, w252) -> (w249:dbl[])
                  n112 = Build Array (concatenate)(w248, w251) -> (w247:dbl[])
                  n113 = Build Array (concatenate)(w258, w257) -> (w256:dbl[][])
                }
                frame 1 {
                }
              }
            }
            "Blade 1 Every Pass" <- w206
            "Blade 3 Every Pass" <- w204
            "Blade 2 Every Pass" <- w205
          }
          frame #1 {
            n114 = Transpose 2D Array(2D array=w289) -> (transposed array=w286:dbl[][])
            "Blade Angles" <- w286
            n115 = Transpose 2D Array(2D array=w288) -> (transposed array=w287:dbl[][])
            "Blade Positions" <- w287
            n116 = for {
              tunnel: w286 -> [w297] mode=indexing
              tunnel: w287 -> [w296] mode=indexing
              tunnel: [w290] -> w285 mode=indexing
              n117 = call <vilib>:"Std Deviation and Variance.vi"("X"=w297) -> ("mean"=w295:dbl, "variance"=w294:dbl)  [unwired: 1 in, 1 out]
              n118 = call <vilib>:"Std Deviation and Variance.vi"("X"=w296) -> ("mean"=w293:dbl, "variance"=w292:dbl)  [unwired: 1 in, 1 out]
              n119 = Build Array(w295, w294, w293, w292) -> (w291:dbl[])
              n120 = Number To Fractional String(number=w291) -> (F-format string=w290:string[])  [unwired: 3 in]
            }
            "Blade Analysis" <- w285
          }
        }
      }
      frame "Phase locked Stats" {
        # "N"
        # "U2T"
        # "UT"
        # "T"
        n121 = while {
          tunnel: w308 -> [w312]
          tunnel: w307 -> [w314]
          tunnel: w302 -> [w329]
          shift-right: [w318] -> _
          shift-left: _ -> [w324]
          tunnel: w303 -> [w311]
          shift-right: [w317] -> _
          shift-left: _ -> [w323]
          shift-right: [w316] -> _
          shift-left: _ -> [w322]
          shift-right: [w315] -> _
          shift-left: _ -> [w321]
          tunnel: w301 -> [w330]
          tunnel: [w320] -> w300
          tunnel: [w319] -> w298
          stop <- TRUE stop-if-true
          n122 = case shown="2, Default" w330 {
            tunnel: w312 -> [_ w342]
            tunnel: w329 -> [_ w341]
            tunnel: [w338 w339] -> w328
            tunnel: [w337 w339] -> w327
            tunnel: [w336 w339] -> w326
            tunnel: [w335 w339] -> w325
            tunnel: w324 -> [w338 _]
            tunnel: w323 -> [w337 _]
            tunnel: w322 -> [w336 _]
            tunnel: w321 -> [w335 _]
            frame 2, Default {
            }
            frame 1 {
              n123 = Array Size(array=w341) -> (size(s)=w340:i32)
              n124 = Initialize Array(0.0, w340, w342) -> (w339:dbl[][])
            }
          }
          n125 = Array Size(array=w311) -> (size(s)=w310:i32)
          n126 = for {
            N: w312 -> [_]
            tunnel: w314 -> [w333]
            tunnel: [w332] -> w313 mode=indexing
            i -> [w334]
            n127 = Multiply(x=w334, y=w333) -> (x*y=w332:dbl)
          }
          "X array" <- w313
          n128 = property on="Channel to Phase lock" class="LstBox (strict)"() -> ("Item Names"=w309:string[])  [unwired: 2 in, 2 out]
          n129 = for {
            tunnel: w312 -> [w372]
            tunnel: w314 -> [_]
            tunnel: w329 -> [w345] mode=indexing
            tunnel: w311 -> [w368]
            tunnel: w328 -> [w357] mode=indexing
            tunnel: [w353] -> w318 mode=indexing
            tunnel: [w352] -> w317 mode=indexing
            tunnel: [w351] -> w316 mode=indexing
            tunnel: [w350] -> w315 mode=indexing
            tunnel: w327 -> [w356] mode=indexing
            tunnel: w326 -> [w355] mode=indexing
            tunnel: w325 -> [w354] mode=indexing
            tunnel: [w360] -> w320 mode=indexing
            tunnel: [w358] -> w319 mode=indexing
            tunnel: w313 -> [w349]
            tunnel: w310 -> [_]
            tunnel: w309 -> [w347]
            i -> [w348]
            # "u^2"
            # "U"
            # "U2T"
            # "UT"
            # "T"
            n130 = To Long Integer(number=w372) -> (32bit integer=w371:i32)
            n131 = Index Array(array=w347, index=w345) -> (element=w346:string)
            n132 = property on="Inst Channels" class="XYGraph (strict)"("Active Plot"=w348, "Plot.Plot Name"=w346) -> ()  [unwired: 2 in, 2 out]
            n133 = local read "WT Revolution Start times"() -> (w376:dbl[])
            n134 = Index Array(array=w368, index=w345) -> (element=w344:T6)
            n135 = Unbundle By Name(w344) -> ("Time (s)"=w370:dbl[], "Eng Values"=w369:dbl[], "Weighting"=w367:dbl[])
            n136 = call "Create_Bin_Indices.vi"("No Of Bins"=w371, "Cycle Start TIme"=w376) -> ("Bin Number"=w374:i32[], "Bin Start Time"=w375:dbl[])
            n137 = for {
              tunnel: w375 -> [w408]
              tunnel: w370 -> [w407] mode=indexing
              shift-right: [w404] -> _
              shift-left: 0 -> [w401]
              tunnel: w374 -> [w405]
              tunnel: [w403] -> w373 mode=indexing
              n138 = Threshold 1D Array(1:w401, 2:w407, 3:w408) -> (0:w406:dbl)
              n139 = Round Toward -Infinity(1:w406) -> (0:w402:dbl)
              n140 = To Long Integer(number=w402) -> (32bit integer=w404:i32)
              n141 = Index Array(array=w405, index=w404) -> (element=w403:i32)
            }
            n142 = for {
              tunnel: w373 -> [w387] mode=indexing
              tunnel: w369 -> [w379] mode=indexing
              tunnel: w367 -> [w378] mode=indexing
              shift-right: [w383] -> w353
              shift-left: w357 -> [w388]
              shift-right: [w382] -> w352
              shift-left: w356 -> [w384]
              shift-right: [w381] -> w351
              shift-left: w355 -> [w385]
              shift-right: [w380] -> w350
              shift-left: w354 -> [w386]
              n143 = in-place {
                in-place-border: w379 -> [w393]
                in-place-border: w378 -> [w396]
                n144 = in-place-array #1(w385, w387) -> (w390:dbl)
                n145 = in-place-array #2(w388, w387) -> (w400:dbl)
                n146 = in-place-array #3(w384, w387) -> (w398:dbl)
                n147 = in-place-array #4(w386, w387) -> (w389:dbl)
                n148 = Add(x=w396, y=w398) -> (x+y=w397:dbl)
                n149 = Multiply(x=w393, y=w396) -> (x*y=w395:dbl)
                n150 = Add(x=w395, y=w390) -> (x+y=w391:dbl)
                n151 = Multiply(x=w393, y=w395) -> (x*y=w394:dbl)
                n152 = Increment(x=w400) -> (x+1=w399:dbl)
                n153 = Add(x=w394, y=w389) -> (x+y=w392:dbl)
                n154 = in-place-array #1(w391) -> (w381:dbl[])  [unwired: 1 out]
                n155 = in-place-array #2(w399) -> (w383:dbl[])  [unwired: 1 out]
                n156 = in-place-array #3(w397) -> (w382:dbl[])  [unwired: 1 out]
                n157 = in-place-array #4(w392) -> (w380:dbl[])  [unwired: 1 out]
              }
            }
            n158 = Divide(x=w350, y=w353) -> (x/y=w364:dbl[])
            n159 = Divide(x=w351, y=w353) -> (x/y=w366:dbl[])
            n160 = Divide(x=w352, y=w353) -> (x/y=w365:dbl[])
            n161 = Divide(x=w364, y=w365) -> (x/y=w363:dbl[])
            n162 = Divide(x=w366, y=w365) -> (x/y=w359:dbl[])
            n163 = Square(x=w359) -> (x^2=w362:dbl[])
            n164 = Subtract(x=w363, y=w362) -> (x-y=w361:dbl[])
            n165 = Bundle(w359, w361) -> (w360:cluster{dbl[], dbl[]})  [unwired: 1 in]
            n166 = Bundle(w349, w359) -> (w358:cluster{dbl[], dbl[]})  [unwired: 1 in]
          }
        }
        "Inst Channels" <- w298
      }
      frame "Cross correlation phase locking" {
        n167 = To Long Integer(number=w411) -> (32bit integer=w410:i32)
        n168 = stacked-sequence {
          seq-local: [w422 _] -> [_ w475]
          seq-local: [w421 _] -> [_ w474]
          tunnel: w414 -> [w426 _]
          tunnel: w413 -> [w425 _]
          tunnel: w412 -> [w424 _]
          tunnel: w410 -> [w423 w473]
          tunnel: w409 -> [_ w470]
          frame #0 {
            n169 = while {
              shift-right: [w439] -> _
              shift-left: _ -> [w438]
              tunnel: w426 -> [w435]
              tunnel: w425 -> [w434]
              tunnel: w424 -> [w433]
              tunnel: w423 -> [w430]
              tunnel: [w428] -> w422
              tunnel: [w427] -> w421
              stop <- TRUE stop-if-true
              n170 = local read "WT Revolution Start times"() -> (w431:dbl[])
              n171 = local read "X array"() -> (w437:dbl[])
              n172 = for {
                tunnel: [w466] -> w439 mode=indexing
                tunnel: w438 -> [w465]
                tunnel: w437 -> [w462]
                tunnel: [w460] -> w428 mode=indexing
                tunnel: "Cross_Corr to Phase Lock" -> [w459] mode=indexing
                tunnel: w435 -> [w458]
                tunnel: w434 -> [w456]
                tunnel: w433 -> [w454]
                tunnel: w431 -> [w450]
                tunnel: w430 -> [w449]
                tunnel: "Time Shift" -> [w446]
                tunnel: [w440] -> w427 mode=indexing
                i -> [w464]
                w451 = 0 items=["nearest", "linear", "spline", "cubic Hermite", "Lagrange"] ("interp. method")
                n173 = Index Array(array=w458, index (row)=w459) -> (element=w457:i32[])  [unwired: 1 in]
                n174 = Index Array(array=w465, index (dim 0)=w464) -> (element=w463:dbl[][])  [unwired: 2 in]
                n175 = Index Array(array=w457) -> (element #1=w453:i32, element #2=w452:i32)  [unwired: 2 in]
                n176 = Index Array(array=w456, index=w453) -> (element=w448:T6)
                n177 = Index Array(array=w454, index=w453) -> (element=w445:T3)
                n178 = Index Array(array=w456, index=w452) -> (element=w455:T6)
                n179 = Index Array(array=w454, index=w452) -> (element=w444:T3)
                n180 = in-place {
                  in-place-border: w446 -> [w469]
                  n181 = in-place-cluster #5(w448) -> ("Time (s)"=w468:dbl[])
                  n182 = Add(x=w469, y=w468) -> (x+y=w467:dbl[])
                  n183 = in-place-cluster #5("Time (s)"=w467) -> (w447:T6)
                }
                n184 = Unbundle By Name(w445) -> ("Inst name"=w443:string)
                n185 = Unbundle By Name(w444) -> ("Inst name"=w442:string)
                n186 = call "Phase_Av_Weighted_Cross_Moments.vi"("AI Cluster 1"=w445, "WT Revolution Start times"=w450, "Time Cluster 1"=w447, "AI Cluster 2"=w444, "Time Cluster 2"=w455, "Shift in"=w463, "interp. method"=w451, "No Of Bins"=w449) -> ("Phase locked uw/u'w'"=w461:dbl[], "Shift out"=w466:dbl[][])  [unwired: 5 in, 1 out]
                n187 = Format Into String(format string="%s & %s", w443, w442) -> (resulting string=w440:string)  [unwired: 2 in, 1 out]
                n188 = Bundle("X array"=w462, "Phase locked uw/u'w'"=w461) -> (w460:T7)  [unwired: 1 in]
              }
              "Cross Chs" <- w428
            }
          }
          frame #1 {
            n189 = local read "Add Phase data to results file"() -> (w471:bool)
            n190 = Compound Arithmetic op=AND(w471, w470) -> (w472:bool)
            n191 = case shown="True" w472 {
              tunnel: w475 -> [_ w478]
              tunnel: w474 -> [_ w477]
              tunnel: w473 -> [_ w476]
              frame False {
              }
              frame True {
                n192 = stacked-sequence {
                  tunnel: w476 -> [w481 _]
                  tunnel: w478 -> [_ w498]
                  tunnel: w477 -> [w479 _]
                  frame #0 {
                    n193 = local read "Plug in titles"() -> (w482:string[])
                    n194 = Divide(x=360, y=w481) -> (x/y=w484:dbl)
                    n195 = Increment(x=w481) -> (x+1=w480:i32)
                    n196 = for {
                      tunnel: w479 -> [w491] mode=indexing
                      tunnel: w484 -> [w490]
                      shift-right: [w487] -> w483
                      shift-left: w482 -> [w489]
                      tunnel: w480 -> [w486]
                      n197 = for {
                        N: w486 -> [_]
                        tunnel: w491 -> [w493]
                        tunnel: w490 -> [w496]
                        tunnel: [w494] -> w488 mode=indexing
                        i -> [w497]
                        n198 = Multiply(x=w496, y=w497) -> (x*y=w492:dbl)
                        n199 = Format Into String(format string="%s:Mean:%.1f Deg:%.1f", w493, w492, w492) -> (resulting string=w494:string)  [unwired: 2 in, 1 out]
                      }
                      n200 = Build Array (concatenate)(w489, w488) -> (w487:string[])
                    }
                    n201 = local write "Plug in titles"(w483) -> ()
                  }
                  frame #1 {
                    n202 = local read "Plug in values"() -> (w500:string[])
                    n203 = for {
                      tunnel: w498 -> [w502] mode=indexing
                      shift-right: [w504] -> w499
                      shift-left: w500 -> [w505]
                      n204 = Unbundle(w502) -> ("Phase locked uw/u'w'"=w501:dbl[])  [unwired: 1 out]
                      n205 = for {
                        tunnel: w501 -> [w506] mode=indexing
                        tunnel: [w507] -> w503 mode=indexing
                        n206 = call "Number_2_string.vi"("number"=w506) -> ("String"=w507:string)  [unwired: 1 in]
                      }
                      n207 = Build Array (concatenate)(w505, w503) -> (w504:string[])
                    }
                    n208 = local write "Plug in values"(w499) -> ()
                  }
                }
              }
            }
          }
        }
      }
      frame "Output WT Statistics" {
        n209 = property on="Turbine to Phase Lock to" class="Ring (strict)"() -> ("Strings []"=w524:string[])  [unwired: 2 in, 2 out]
        n210 = for {
          shift-right: [w551] -> w516
          shift-left: "WT" -> [w552]
          tunnel: w524 -> [w542] mode=indexing
          tunnel: [w547] -> w523 mode=indexing
          n211 = String Subset(string=w542, offset (0)=6, length (rest)=1 ("length (rest)")) -> (substring=w538:string)
          n212 = String Subset(string=w542, offset (0)=7, length (rest)=1 ("length (rest)")) -> (substring=w537:string)
          n213 = Equal?(x=")", y=w537) -> (x = y?=w540:bool)
          n214 = case shown="True" w540 {
            tunnel: [w554 w557] -> w539
            tunnel: w538 -> [w556 w557]
            tunnel: w537 -> [w555 _]
            frame False {
              n215 = Concatenate Strings(w556, w555) -> (w554:string)
            }
            frame True {
            }
          }
          n216 = Equal?(x=")", y=w538) -> (x = y?=w548:bool)
          n217 = Select(t="1", s=w548, f=w539) -> (s? t:f=w547:string)
          n218 = Concatenate Strings(w552, "_", w547) -> (w551:string)
        }
        "WT Numbers" <- w523
        n219 = local read "All WTs"() -> (w522:dbl[][])
        n220 = Build Array(w516) -> (w514:string[])
        n221 = Build Array("Wind:Turbines:Logged") -> (w515:string[])
        n222 = for {
          tunnel: w522 -> [w569] mode=indexing
          shift-right: [w563] -> w512
          shift-left: w514 -> [w564]
          shift-right: [w558] -> w513
          shift-left: w515 -> [w561]
          tunnel: string[] ["WT_%s:Hub_RPM:Mean", "WT_%s:Hub_RPM:St_Dev", "WT_%s:Hub_RPM:Max-Min", "WT_%s:Number_of:Revs"] ("Plug in titles") -> [w562]
          tunnel: w523 -> [w559] mode=indexing
          n223 = Index Array(array=w569, index=0) -> (element=w568:dbl)
          n224 = Index Array(array=w569, index=1) -> (element=w567:dbl)
          n225 = Index Array(array=w569, index=2) -> (element=w566:dbl)
          n226 = Index Array(array=w569, index=3) -> (element=w565:dbl)
          n227 = for {
            tunnel: w562 -> [w580] mode=indexing
            tunnel: [w579] -> w560 mode=indexing
            tunnel: w559 -> [w578]
            n228 = Format Into String(format string=w580, w578) -> (resulting string=w579:string)  [unwired: 2 in, 1 out]
          }
          n229 = call "Number_2_string.vi"("number"=w568) -> ("String"=w576:string)  [unwired: 1 in]
          n230 = call "Number_2_string.vi"("number"=w567) -> ("String"=w577:string)  [unwired: 1 in]
          n231 = call "Number_2_string.vi"("number"=w566) -> ("String"=w575:string)  [unwired: 1 in]
          n232 = Number To Decimal String(number=w565) -> (decimal integer string=w574:string)  [unwired: 1 out]
          n233 = Build Array (concatenate)(w564, w576, w577, w575, w574) -> (w563:string[])
          n234 = Build Array (concatenate)(w561, w560) -> (w558:string[])
        }
        n235 = Decimal String To Number(string=w523) -> (number=w520:i32[])  [unwired: 2 in, 1 out]
        n236 = Index Array(array=w522, index (col)=0 ("disabled index (col)")) -> (element=w519:dbl[])  [unwired: 1 in]
        n237 = local read "Laser Disp Index"() -> (w534:i32)
        n238 = Bundle(w520, "All WTs"=w519) -> (→"Turbine RPMs":cluster{i32[], "All WTs":dbl[]})  [unwired: 1 in]
        n239 = Greater Or Equal To 0?(x=w534) -> (x >= 0?=w533:bool)
        n240 = local read "Plug in values"() -> (w510:string[])
        n241 = local read "Plug in titles"() -> (w511:string[])
        n242 = Build Array (concatenate)(w513, w511) -> (→"Plug in titles":string[])
        n243 = Build Array (concatenate)(w512, w510) -> (→"Plug in values":string[])
        n244 = Select(t="Laser Displacement Analysis", s=w533, f="Get Last Block info") -> (s? t:f=w532:string)
      }
      frame "Laser Displacement Analysis" {
        # "L"
        # "S"
        # "R"
        # "D^2"
        # "D"
        n245 = stacked-sequence {
          seq-local: [_ w599 _ _ _ _ _] -> [_ _ w617 _ _ _ _]
          seq-local: [_ _ w618 _ _ _ _] -> [_ _ _ _ w684 _ _]
          seq-local: [w592 _ _ _ _ _ _] -> [_ _ _ _ w680 _ _]
          seq-local: [w593 _ _ _ _ _ _] -> [_ _ _ _ w679 _ _]
          seq-local: [_ _ _ w654 _ _ _] -> [_ _ _ _ w672 _ _]
          seq-local: [_ _ _ w649 _ _ _] -> [_ _ _ _ w671 _ _]
          seq-local: [_ _ _ w652 _ _ _] -> [_ _ _ _ w670 _ _]
          seq-local: [w593 _ _ _ _ _ _] -> [_ w600 _ _ _ _ _]
          tunnel: w591 -> [_ _ _ _ _ _ _]
          tunnel: w590 -> [_ _ _ _ _ _ _]
          tunnel: w589 -> [_ _ _ w650 w673 _ _]
          tunnel: w588 -> [_ _ _ _ _ w758 w796]
          tunnel: [_ _ _ _ _ TRUE _] -> w587
          tunnel: [_ _ _ _ _ "Get Last Block info" _] -> w586
          tunnel: w582 -> [w596 w603 _ _ _ _ _]
          tunnel: w581 -> [_ _ _ w668 _ _ _]
          frame #0 {
            n246 = local read "Laser Phase lock index"() -> (w594:i32)
            n247 = Index Array(array=w596, index=w594) -> (element=w595:cluster{dbl[], dbl[]})
            n248 = Unbundle(w595) -> (w593:dbl[], w592:dbl[])
            n249 = Build Array (concatenate)(w593, w593, 0.0) -> ()  [unwired: 1 out]
            n250 = Build Array (concatenate)(w592, w592, 0.0) -> ()  [unwired: 1 out]
          }
          frame #1 {
            n251 = local read "Laser Status Index"() -> (w602:i32)
            n252 = Less Than 0?(x=w602) -> (x < 0?=w601:bool)
            n253 = case shown="True" w601 {
              tunnel: w603 -> [w609 _]
              tunnel: w600 -> [_ w616]
              tunnel: [w605 w611] -> w599
              frame False {
                n254 = local read "L Status Phase lock index"() -> (w608:i32)
                n255 = Index Array(array=w609, index=w608) -> (element=w610:cluster{dbl[], dbl[]})
                n256 = Unbundle(w610) -> (w604:dbl[])  [unwired: 1 out]
                n257 = Build Array (concatenate)(w604, w604, 0.0) -> ()  [unwired: 1 out]
                n258 = Greater?(x=w604, y=0.4) -> (0:w605:bool[])
              }
              frame True {
                n259 = Greater?(x=w616, y=-5) -> (0:w612:bool[])
                n260 = Build Array (concatenate)(w612, w612, FALSE) -> (w613:bool[])
                n261 = Not(x=w613) -> (.not. x?=w611:bool[])
              }
            }
          }
          frame #2 {
            n262 = Index Array(array=w617, index=0) -> (element=w620:bool)
            n263 = for {
              tunnel: w617 -> [w627] mode=indexing
              shift-right: [w627] -> _
              shift-left: w620 -> [w622]
              shift-right: [w624] -> w618
              shift-left: i32[] [] -> [w625]
              i -> [w626]
              n264 = Not Equal?(x=w627, y=w622) -> (x != y?=w623:bool)
              n265 = case shown="True" w623 {
                tunnel: w626 -> [_ w634]
                tunnel: w625 -> [w628 w632]
                tunnel: [w628 w633] -> w624
                tunnel: w622 -> [_ w629]
                frame False {
                }
                frame True {
                  n266 = Array Size(array=w632) -> (size(s)=w631:i32)
                  n267 = Equal To 0?(x=w631) -> (x = 0?=w630:bool)
                  n268 = case shown="True" w630 {
                    tunnel: w634 -> [w635 w641]
                    tunnel: w632 -> [w637 w640]
                    tunnel: [w636 w639] -> w633
                    tunnel: w629 -> [_ w638]
                    frame False {
                      n269 = Build Array (concatenate)(w637, w635) -> (w636:i32[])
                    }
                    frame True {
                      n270 = case shown="False" w638 {
                        tunnel: w641 -> [_ w645]
                        tunnel: w640 -> [w642 w644]
                        tunnel: [w642 w643] -> w639
                        frame False {
                        }
                        frame True {
                          n271 = Build Array (concatenate)(w644, w645) -> (w643:i32[])
                        }
                      }
                    }
                  }
                }
              }
            }
          }
          frame #3 {
            n272 = local read "Laser Disp Index"() -> (w667:i32)
            n273 = Index Array(array=w668, index=w667) -> (element=w669:T3)
            n274 = Unbundle By Name(w669) -> ("Y"=w660:dbl)
            n275 = Absolute Value(x=w660) -> (abs(x)=w654:dbl)
            n276 = formula code="S=(0.0001*R*R) -0.0619*R+7.7094;"("R"=w654) -> ("S"=w648:dbl)
            n277 = Divide(x=10, y=w654) -> (x/y=w665:dbl)
            n278 = Inverse Tangent(1:w665) -> (0:w664:dbl)
            n279 = Divide(x=w664, y=3.141592653589793) -> (x/y=w662:dbl)
            n280 = Max & Min(x=w648, y=0.0) -> (max(x,y)=w646:dbl)  [unwired: 1 out]
            n281 = Divide(x=w646, y=w654) -> (x/y=w655:dbl)
            n282 = Inverse Tangent(1:w655) -> (0:w656:dbl)
            n283 = Divide(x=w656, y=3.141592653589793) -> (x/y=w658:dbl)
            n284 = Multiply(x=w662, y=180.0) -> (x*y=w651:dbl)
            n285 = Multiply(x=w658, y=180.0) -> (x*y=w653:dbl)
            n286 = Divide(x=w653, y=w650) -> (x/y=w652:dbl)
            n287 = Divide(x=w651, y=w650) -> (x/y=w649:dbl)
          }
          frame #4 {
            w674 = 360.0 ("y")
            n288 = Divide(x="Start Cut Deg", y=w673) -> (x/y=w686:dbl)
            n289 = Divide(x="End Cut Deg", y=w673) -> (x/y=w687:dbl)
            n290 = To Long Integer(number=w686) -> (32bit integer=w682:i32)
            n291 = To Long Integer(number=w687) -> (32bit integer=w685:i32)
            n292 = Add(x=w682, y=w685) -> (x+y=w681:i32)
            n293 = Divide(x=w673, y=w674) -> (x/y=w678:dbl)
            n294 = Multiply(x=w678, y=6.283185307179586) -> (x*y=w677:dbl)
            n295 = Multiply(x=w677, y=w672) -> (x*y=w675:dbl)
            n296 = for {
              N: 3 -> [_]
              tunnel: w679 -> [w725]
              tunnel: w684 -> [w722]
              tunnel: w682 -> [w692]
              tunnel: w681 -> [w718]
              tunnel: w675 -> [w717]
              tunnel: w680 -> [w709]
              tunnel: w674 -> [w702]
              tunnel: w673 -> [w696]
              tunnel: w671 -> [w694]
              tunnel: w670 -> [w690]
              i -> [w716]
              n297 = Multiply(x=w716, y=2) -> (x*y=w720:i32)
              n298 = Increment(x=w720) -> (x+1=w719:i32)
              n299 = Index Array(array=w722, index=w720) -> (element=w727:i32)
              n300 = Index Array(array=w722, index=w719) -> (element=w728:i32)
              n301 = Subtract(x=w728, y=w727) -> (x-y=w726:i32)
              n302 = Add(x=w690, y=w692) -> (x+y=w691:dbl)
              n303 = Add(x=w727, y=w691) -> (x+y=w712:dbl)
              n304 = Subtract(x=w726, y=w718) -> (x-y=w695:i32)
              n305 = Max & Min(x=w695, y=w694) -> (min(x,y)=w693:dbl)  [unwired: 1 out]
              n306 = Array Subset(array=w709, index=w712, length=w693) -> (w700:dbl[])
              n307 = call-poly <vilib>:"Mean.vi"("X"=w700) -> ("mean"=w699:dbl)  [unwired: 1 out]
              n308 = Multiply(x=2.0, y=w699) -> (x*y=w697:dbl)
              n309 = call "Top_and_Tail_ph.vi"("Array in"=w700, "Threshold"=w697) -> ("Length"=w707:i32, "Start Index"=w711:i32)
              n310 = Add(x=w712, y=w711) -> (x+y=w708:dbl)
              n311 = Array Subset(array=w709, index=w708, length=w707) -> (w710:dbl[])
              n312 = call-poly <vilib>:"Mean.vi"("X"=w710) -> ("mean"=w713:dbl)  [unwired: 1 out]
              n313 = Array Subset(array=w725, index=w708, length=w707) -> (w715:dbl[])
              n314 = Array Size(array=w715) -> (size(s)=w724:i32)
              n315 = for {
                N: w724 -> [_]
                tunnel: w717 -> [w755]
                tunnel: [w753] -> w723 mode=indexing
                i -> [w754]
                n316 = Multiply(x=w754, y=w755) -> (x*y=w753:dbl)
              }
              n317 = call <vilib>:"Linear Fit.vi"("Y"=w715, "X"=w723) -> ("slope"=w706:dbl)  [unwired: 9 in, 4 out]
              n318 = call-poly <vilib>:"Mean.vi"("X"=w715) -> ("mean"=w714:dbl)  [unwired: 1 out]
              n319 = Inverse Tangent(1:w706) -> (0:w705:dbl)
              n320 = Divide(x=w705, y=6.283185307179586) -> (x/y=w703:dbl)
              n321 = Multiply(x=w703, y=w702) -> (x*y=w701:dbl)
              n322 = case shown="0, Default" w716 {
                tunnel: w715 -> [w732 w739 w746]
                tunnel: w706 -> [w736 w743 w751]
                tunnel: w714 -> [w735 w744 w752]
                tunnel: w710 -> [_ _ _]
                tunnel: w713 -> [w734 w742 w750]
                tunnel: w701 -> [w733 w741 w749]
                tunnel: w696 -> [w729 w740 w747]
                frame 0, Default {
                  n323 = Bundle(0.0, "Angular Step"=w729, w732) -> (→"Mean Blade 1":cluster{dbl, "Angular Step":dbl, dbl[]})  [unwired: 1 in]
                  "slope 1" <- w736
                  "Av Disp 1" <- w735
                  "Av Variance 1" <- w734
                  "Angle 1" <- w733
                }
                frame 1 {
                  n324 = Bundle(0.0, "Angular Step"=w740, w739) -> (→"Mean Blade 2":cluster{dbl, "Angular Step":dbl, dbl[]})  [unwired: 1 in]
                  "Av Disp 2" <- w744
                  "slope 2" <- w743
                  "Av Variance 2" <- w742
                  "Angle 2" <- w741
                }
                frame 2 {
                  n325 = Bundle(0.0, "Angular Step"=w747, w746) -> (→"Mean Blade 3":cluster{dbl, "Angular Step":dbl, dbl[]})  [unwired: 1 in]
                  "Av Disp 3" <- w752
                  "slope 3" <- w751
                  "Av Variance 3" <- w750
                  "Angle 3" <- w749
                }
              }
            }
          }
          frame #5 {
            n326 = case shown="True" w758 {
              frame False {
              }
              frame True {
                n327 = for {
                  N: 3 -> [_]
                  tunnel: [w789] -> w780 mode=indexing
                  tunnel: [w788] -> w779 mode=indexing
                  tunnel: [w787] -> w778 mode=indexing
                  tunnel: [w786] -> w762 mode=indexing
                  i -> [w795]
                  n328 = Increment(x=w795) -> (x+1=w794:i32)
                  n329 = Format Into String(format string="Blade %d:", w794) -> (resulting string=w785:string)  [unwired: 2 in, 1 out]
                  n330 = Concatenate Strings(w785, "Angle:") -> (w786:string)
                  n331 = Concatenate Strings(w785, "Slope:") -> (w789:string)
                  n332 = Concatenate Strings(w785, "Average:X") -> (w788:string)
                  n333 = Concatenate Strings(w785, "Variance of:X") -> (w787:string)
                }
                n334 = local read "Av Variance 1"() -> (w769:dbl)
                n335 = local read "Av Variance 2"() -> (w768:dbl)
                n336 = local read "Av Variance 3"() -> (w767:dbl)
                n337 = local read "Av Disp 1"() -> (w772:dbl)
                n338 = local read "Av Disp 2"() -> (w771:dbl)
                n339 = local read "Av Disp 3"() -> (w770:dbl)
                n340 = local read "Angle 3"() -> (w761:dbl)
                n341 = local read "slope 1"() -> (w775:dbl)
                n342 = local read "slope 2"() -> (w774:dbl)
                n343 = local read "slope 3"() -> (w773:dbl)
                n344 = local read "Angle 1"() -> (w760:dbl)
                n345 = local read "Angle 2"() -> (w759:dbl)
                n346 = Build Array(w760, w759, w761, w775, w774, w773, w772, w771, w770, w769, w768, w767) -> (w766:dbl[])
                n347 = local read "Plug in values"() -> (w765:string[])
                n348 = local read "Plug in titles"() -> (w777:string[])
                n349 = for {
                  tunnel: w766 -> [w783] mode=indexing
                  tunnel: [w782] -> w764 mode=indexing
                  n350 = call "Number_2_string.vi"("number"=w783) -> ("String"=w782:string)  [unwired: 1 in]
                }
                n351 = Build Array (concatenate)(w777, w762, w780, w779, w778) -> (w776:string[])
                n352 = Build Array (concatenate)(w765, w764) -> (w763:string[])
                n353 = local write "Plug in titles"(w776) -> ()
                n354 = local write "Plug in values"(w763) -> ()
              }
            }
          }
          frame #6 {
            n355 = case shown="True" w796 {
              frame False {
              }
              frame True {
                n356 = local read "Blade Analysis"() -> (w800:string[][])
                n357 = for {
                  tunnel: [w805] -> w803 mode=concatenating
                  tunnel: w800 -> [w804] mode=indexing
                  tunnel: [w804] -> w797 mode=concatenating
                  i -> [w817]
                  n358 = Increment(x=w817) -> (x+1=w816:i32)
                  n359 = Format Into String(format string="Blade %d:", w816) -> (resulting string=w811:string)  [unwired: 2 in, 1 out]
                  n360 = Concatenate Strings(w811, "Angle:Degrees") -> (w809:string)
                  n361 = Concatenate Strings(w811, "Angle:Variance") -> (w808:string)
                  n362 = Concatenate Strings(w811, "Position:(mm)") -> (w807:string)
                  n363 = Concatenate Strings(w811, "Position:Variance") -> (w806:string)
                  n364 = Build Array(w809, w808, w807, w806) -> (w805:string[])
                }
                n365 = local read "Plug in titles"() -> (w802:string[])
                n366 = local read "Plug in values"() -> (w799:string[])
                n367 = Build Array (concatenate)(w802, w803) -> (w801:string[])
                n368 = Build Array (concatenate)(w799, w797) -> (w798:string[])
                n369 = local write "Plug in values"(w798) -> ()
                n370 = local write "Plug in titles"(w801) -> ()
              }
            }
          }
        }
      }
      frame "Get Last Block info" {
        n371 = case shown="\"Take New Data\"" w825 {
          tunnel: [w826 "Post Process"] -> w824
          tunnel: [w830 TRUE ("Processing last block?")] -> w823
          tunnel: w822 -> [w830 _]
          frame "Take New Data" {
            n372 = Select(t="Change Dem Volts", s="Change Dem Voltages?", f="Post Process") -> (s? t:f=w826:string)
          }
          frame "Post Process Raw Data File" {
          }
        }
      }
      frame "Change Dem Volts" {
        n373 = local read "WT Numbers"() -> (w835:string[])
        n374 = local read "All WTs"() -> (w861:dbl[][])
        n375 = for {
          N: 11 -> [_]
          tunnel: w865 -> [w891]
          tunnel: [w890] -> w864 mode=indexing
          tunnel: [w889] -> w847 mode=indexing
          tunnel: w861 -> [w887] mode=indexing
          tunnel: [w886] -> w859 mode=indexing
          tunnel: [w885] -> w841
          tunnel: w840 -> [w884]
          tunnel: w835 -> [w883] mode=indexing
          i -> [w892]
          n376 = Increment(x=w892) -> (x+1=w885:i32)
          n377 = Format Into String(format string=w891, w883) -> (resulting string=w889:string)  [unwired: 2 in, 1 out]
          n378 = Format Into String(format string=w884, w883) -> (resulting string=w890:string)  [unwired: 2 in, 1 out]
          n379 = Index Array(array=w887, index=0) -> (element=w886:dbl)
        }
        n380 = Build Array (concatenate)(w864, w847) -> (w863:string[])
        n381 = call "Get_Current_Scan_client.vi"("ADAM Ch Names"=w863) -> ("Numerical Values"=w862:dbl[])  [unwired: 3 out]
        n382 = Split 1D Array(array=w862, index=w841) -> (first subarray=w860:dbl[], second subarray=w858:dbl[])
        n383 = Divide(x=w860, y=w859) -> (x/y=w850:dbl[])
        n384 = In Range and Coerce(upper limit=1.05, x=w850, lower limit=0.95) -> (coerced(x)=w849:dbl[], In Range?=w848:bool[])
        n385 = Multiply(x=w849, y=w858) -> (x*y=w853:dbl[])
        n386 = In Range and Coerce(upper limit=9.9, x=w853, lower limit=0.0) -> (coerced(x)=w846:dbl[])  [unwired: 1 out]
        n387 = for {
          shift-right: [w873] -> w844
          shift-left: string[] [] -> [w874]
          shift-right: [w871] -> w845
          shift-left: dbl[] [] -> [w872]
          tunnel: w848 -> [w868] mode=indexing
          tunnel: w847 -> [w870] mode=indexing
          tunnel: w846 -> [w869] mode=indexing
          tunnel: "Allow large changes?" -> [w866]
          n388 = Or(x=w866, y=w868) -> (x .or. y?=w867:bool)
          n389 = case shown="False" w867 {
            tunnel: w874 -> [w876 w882]
            tunnel: [w876 w881] -> w873
            tunnel: w872 -> [w875 w880]
            tunnel: [w875 w879] -> w871
            tunnel: w870 -> [_ w878]
            tunnel: w869 -> [_ w877]
            frame False {
            }
            frame True {
              n390 = Build Array (concatenate)(w882, w878) -> (w881:string[])
              n391 = Build Array (concatenate)(w880, w877) -> (w879:dbl[])
            }
          }
        }
        n392 = call "ASYNC_Adam_client.vi"("Values"=w845, "Channel Names"=w844) -> ()  [unwired: 2 out]
      }
      frame "Post Process" {
        n393 = Compound Arithmetic op=AND("Add Phase data to results file", w899) -> (w898:bool)
        n394 = case shown="True" w898 {
          tunnel: w897 -> [_ w905]
          tunnel: w893 -> [_ w904]
          frame False {
          }
          frame True {
            n395 = stacked-sequence {
              tunnel: w905 -> [w907 _]
              tunnel: w904 -> [_ w933]
              frame #0 {
                n396 = local read "Channel to Phase lock"() -> (w914:i32[])
                n397 = property on="Channel to Phase lock" class="LstBox (strict)"() -> ("Item Names"=w913:string[])  [unwired: 2 in, 2 out]
                n398 = local read "Plug in titles"() -> (w908:string[])
                n399 = Divide(x=360, y=w907) -> (x/y=w910:dbl)
                n400 = Increment(x=w907) -> (x+1=w906:dbl)
                n401 = for {
                  tunnel: w913 -> [w932]
                  tunnel: w914 -> [w931] mode=indexing
                  tunnel: [w930] -> w912 mode=indexing
                  n402 = Index Array(array=w932, index=w931) -> (element=w930:string)
                }
                n403 = for {
                  tunnel: w912 -> [w921] mode=indexing
                  tunnel: w910 -> [w920]
                  shift-right: [w917] -> w909
                  shift-left: w908 -> [w919]
                  tunnel: w906 -> [w915]
                  n404 = for {
                    N: w915 -> [_]
                    tunnel: w921 -> [w924]
                    tunnel: w920 -> [w928]
                    tunnel: [w926] -> w918 mode=indexing
                    tunnel: [w923] -> w916 mode=indexing
                    i -> [w929]
                    n405 = Multiply(x=w928, y=w929) -> (x*y=w922:dbl)
                    n406 = Format Into String(format string="%s:Mean:%.1f Deg:%.1f", w924, w922, w922) -> (resulting string=w926:string)  [unwired: 2 in, 1 out]
                    n407 = Format Into String(format string="%s:Variance:%.1f Deg:%.1f", w924, w922, w922) -> (resulting string=w923:string)  [unwired: 2 in, 1 out]
                  }
                  n408 = Build Array (concatenate)(w919, w918, w916) -> (w917:string[])
                }
                n409 = local write "Plug in titles"(w909) -> ()
              }
              frame #1 {
                n410 = local read "Plug in values"() -> (w935:string[])
                n411 = for {
                  tunnel: w933 -> [w938] mode=indexing
                  shift-right: [w941] -> w934
                  shift-left: w935 -> [w942]
                  n412 = Unbundle(w938) -> (w936:dbl[], w937:dbl[])
                  n413 = for {
                    tunnel: w936 -> [w945] mode=indexing
                    tunnel: [w946] -> w940 mode=indexing
                    tunnel: w937 -> [w943] mode=indexing
                    tunnel: [w944] -> w939 mode=indexing
                    n414 = call "Number_2_string.vi"("number"=w945) -> ("String"=w946:string)  [unwired: 1 in]
                    n415 = call "Number_2_string.vi"("number"=w943) -> ("String"=w944:string)  [unwired: 1 in]
                  }
                  n416 = Build Array (concatenate)(w942, w940, w939) -> (w941:string[])
                }
                n417 = local write "Plug in values"(w934) -> ()
              }
            }
          }
        }
        n418 = Compound Arithmetic op=AND("Save Phase averaged Profiles", w899) -> (w901:bool)
      }
      frame "Check Folder Name" {
        n419 = File/Directory Info(path="Output Directory") -> (error out=w955:errorcluster)  [unwired: 1 in, 6 out]
        n420 = Empty String/Path?(string/path="Output Directory") -> (empty?=w957:bool)
        n421 = Unbundle By Name(w955) -> ("status"=w956:bool)
        n422 = Or(x=w957, y=w956) -> (x .or. y?=w958:bool)
        n423 = case shown="True" w958 {
          tunnel: [w961 w967] -> w951
          tunnel: "Output Directory" -> [w961 w965]
          tunnel: [FALSE ("cancelled") w962] -> w953
          frame False {
          }
          frame True {
            n424 = Strip Path(path=w965) -> (stripped path=w964:path, name=w963:string)
            n425 = File Dialog(7:"Please Select a new or existing Results folder" ("prompt"), 9:w963, 11:w964) -> (1:w962:bool, 3:w967:path)  [unwired: 1 in, 5 out]
          }
        }
        n426 = local write "Output Directory"(w951) -> ()
        n427 = Not(x=w953) -> (.not. x?=w952:bool)
      }
      frame "Save Phase locked data" {
        n428 = global read "Meas_global.vi" "Raw data file"() -> (w974:path)
        n429 = stacked-sequence {
          seq-local: [_ w1004 _ _] -> [_ _ _ w1062]
          seq-local: [w982 _ _ _] -> [_ _ _ w1063]
          seq-local: [_ _ w1019 _] -> [_ _ _ w1061]
          seq-local: [w977 _ _ _] -> [_ _ w1018 _]
          tunnel: w975 -> [_ _ _ _]
          tunnel: w974 -> [w981 _ _ w1067]
          tunnel: w970 -> [w980 _ _ _]
          tunnel: w969 -> [_ _ w1017 _]
          frame #0 {
            w983 = "\r\n"
            n430 = for {
              tunnel: w980 -> [w988] mode=indexing
              tunnel: [w986] -> w979 mode=indexing
              tunnel: [w987] -> w978 mode=indexing
              n431 = Unbundle(w988) -> (w986:dbl[], w987:dbl[])
            }
            n432 = call "Read_RD_Ch_header.vi"("Raw data file"=w981) -> ("Ch string"=w985:string)  [unwired: 3 out]
            n433 = Concatenate Strings(w983, "*****This is a many rows per single point file*****", w983, w985) -> (w982:string)
            n434 = Build Array (concatenate)(w979, w978) -> (w977:dbl[][])
          }
          frame #1 {
            w990 = "\r\n"
            n435 = local read "Channel to Phase lock"() -> (w1006:i32[])
            n436 = property on="Channel to Phase lock" class="LstBox (strict)"() -> ("Item Names"=w1005:string[])  [unwired: 2 in, 2 out]
            n437 = Initialize Array("", 10) -> (w1007:string[])
            n438 = call "Asterisk_header.vi"("Channel names"=w1007) -> ("Header string"=w989:string)
            n439 = for {
              tunnel: w1006 -> [w1015] mode=indexing
              tunnel: w1005 -> [w1014]
              tunnel: [w1013] -> w1002 mode=indexing
              tunnel: ["Mean" ("format string")] -> w1000 mode=indexing
              tunnel: ["Variance" ("format string")] -> w999 mode=indexing
              tunnel: [""] -> w997 mode=indexing
              n440 = Index Array(array=w1014, index=w1015) -> (element=w1013:string)
            }
            n441 = Build Array (concatenate)("Rotor", w1002, w1002) -> (w996:string[])
            n442 = Build Array (concatenate)("Angle", w1000, w999) -> (w995:string[])
            n443 = Build Array (concatenate)("(deg)", w997, w997) -> (w994:string[])
            n444 = Build Array(w996, w995, w994) -> (w993:string[][])
            n445 = Array To Spreadsheet String(array=w993, 3:"%s" ("format string")) -> (spreadsheet string=w991:string)  [unwired: 1 out]
            n446 = Concatenate Strings(w990, w989, w991, w990) -> (w1004:string)
          }
          frame #2 {
            n447 = Array Size(array=w1018) -> (size(s)=w1020:i32[])
            n448 = Index Array(array=w1020, index=0) -> (element=w1025:i32)
            n449 = Index Array(array=w1020, index=1) -> (element=w1021:i32)
            n450 = Decrement(x=w1025) -> (x-1=w1026:i32)
            n451 = for {
              N: w1021 -> [_]
              shift-right: [w1042] -> w1019
              shift-left: "" -> [w1037]
              tunnel: "Separation Character" -> [w1034]
              tunnel: w1018 -> [w1040]
              tunnel: w1026 -> [w1036]
              tunnel: w1017 -> [w1031]
              tunnel: [w1027] -> _ mode=indexing
              i -> [w1033]
              n452 = Divide(x=w1031, y=2.0) -> (x/y=w1029:dbl)
              n453 = Multiply(x=w1033, y=w1031) -> (x*y=w1028:dbl)
              n454 = Index Array(array=w1040, index (col)=w1033) -> (element=w1039:dbl[])  [unwired: 1 in]
              n455 = Add(x=w1028, y=w1029) -> (x+y=w1027:dbl)
              n456 = call "Number_2_string.vi"("number"=w1027) -> ("String"=w1032:string)  [unwired: 1 in]
              n457 = Concatenate Strings(w1032, w1034) -> (w1035:string)
              n458 = for {
                shift-right: [w1050] -> w1038
                shift-left: w1035 -> [w1051]
                tunnel: w1034 -> [w1049]
                tunnel: w1039 -> [w1045] mode=indexing
                tunnel: w1036 -> [w1047]
                i -> [w1048]
                n459 = Equal?(x=w1048, y=w1047) -> (x = y?=w1046:bool)
                n460 = call "Number_2_string.vi"("precision"="Precision", "number"=w1045) -> ("String"=w1044:string)
                n461 = case shown="False" w1046 {
                  tunnel: w1051 -> [w1055 w1058]
                  tunnel: w1044 -> [w1054 w1057]
                  tunnel: [w1053 w1056] -> w1050
                  tunnel: w1049 -> [w1052 _]
                  frame False {
                    n462 = Concatenate Strings(w1055, w1054, w1052) -> (w1053:string)
                  }
                  frame True {
                    n463 = Concatenate Strings(w1058, w1057) -> (w1056:string)
                  }
                }
              }
              n464 = Concatenate Strings(w1037, w1038, "\r\n") -> (w1042:string)
            }
          }
          frame #3 {
            w1059 = FALSE  # append to file? (new file:F)
            n465 = Strip Path(path=w1067) -> (name=w1065:string)  [unwired: 1 out]
            n466 = local read "Output Directory"() -> (w1066:path)
            n467 = Build Path(base path=w1066, name or relative path=w1065) -> (appended path=w1064:path)
            n468 = Concatenate Strings(w1063, w1062, w1061) -> (w1060:string)
            n469 = call "Write_File_Simple.vi"("append to file? (new file:F)"=w1059, "character string"=w1060, "file path"=w1064) -> ()  [unwired: 2 out]
          }
        }
      }
    }
  }
